vi "Pick&Place_ladder_tang.vi"() -> ()   [LabVIEW 2016]
uses:
  WTF is this.ctl
  Classes/Controllers/I-O/Copy of NI-DAQ Folder/NI-DAQ.lvclass
  D:/INTT/V1/Classes/Controllers/I-O/Copy of I-O Folder/I-O.lvclass
  Classes/Controllers/Dispenser/Copy of Ultimus V2 Folder/Ultimus V2.lvclass
  <vilib>/Analysis/coordinate.llb/2D Cartesian Coordinate Rotation (Scalar).vi
  <vilib>/Utility/file.llb/Read Delimited Spreadsheet (DBL).vi
  <vilib>/Utility/file.llb/Write Delimited Spreadsheet (DBL).vi
  Classes/Controllers/Motion/Copy of Motion Folder/Motion.lvclass
  Classes/Controllers/Camera/Copy of Controller Folder/Controller.lvclass
  <vilib>/Analysis/NI_AALPro.lvlib
  Classes/Controllers/I-O/Copy of I-O Folder/I-O.lvclass
panel:
  out "HDI center positions":dbl[][](array[numeric])=[[459.92445114002015, 980.2358762511564, 78.77350133595746, 0.0015214873297426886]]
  out "x+y":dbl[](array[numeric])
  in  "pick &place module":i32=1
  in  "txt switch":bool
  in  "offset":dbl[][](array[numeric])=[[0.0, 0.0, 0.0, 0.0], [0.0, 0.0, 0.0, 0.0]]
  out "HPoS_CT":dbl[][](array[numeric]) format="%#_8g"
  out "chip distance by OGP":dbl format="%#_8g"
  out "displacement":dbl[](array[numeric])
  out "gantry position test":dbl[](array[numeric])
  out "stave target position":dbl[](array[numeric])
  out "chip distance by gantry":dbl format="%#_8g"
  out "after SL":dbl[](array[numeric]) format="%#_8g"
  out "after SR":dbl[](array[numeric]) format="%#_8g"
  out "after NL":dbl[](array[numeric]) format="%#_8g"
  out "S chip":dbl[](array[numeric]) format="%#_8g"
  out "N chip":dbl[](array[numeric]) format="%#_8g"
  in  "file path (dialog if empty) 2":path=path "C:/Users/PAGANIS/Desktop/shih cheng wei/OGP/test1-2.txt"
  out "bless from OGP !!! Center of  stave":dbl[](array[numeric])
  out "bless from OGP !! measured stave size":dbl[](array[numeric])
  in  "Bless from OGP":bool
  out "FROM Detail !!! Center of module on stave":dbl[](array[numeric])
  out "FROM Detail !! measured stave size":dbl[](array[numeric])
  in  "Align Stave in detail":bool
  in  "check height?":bool
  in  "Uttimus presssure":i64=10
  out "Status":bool
  out "measured HDI top-left position":dbl[][](array[numeric])
  in  "HDI vacuum channel":i32=18
  in  "vacuum":bool=TRUE
  in  "HDI vacuum":bool
  out "measured stave size":dbl[](array[numeric])
  out "Stave mark":dbl[][](array[numeric])
  out "Center of module on stave":dbl[](array[numeric])
  out "Center of HDI from alignment mark":dbl[](array[numeric])
  out "Measured HDI size":dbl[][](array[numeric])
  out "module positions on stave":T1[][](array[typedef])
  in  "Default Stave dimension":dbl[](array[numeric])=[34.0, 472.0, -0.335295, -0.000320234]
  in  "Default Stave upper left mark":dbl[](array[numeric])=[584.376, 675.576, 70.9882, 0.000840064]
  out "Needle parking position":dbl[](array[numeric])
  in  "Uppler / Lower Stave":bool=TRUE
  out "Gantry current position":dbl[](array[numeric])
  in  "READ Position":bool
  in  "Needle Height Compenstation\n(glue gap)":dbl=0.33
  in  "Needle Alignment":bool
  in  "Parking position":dbl[](array[numeric])=[625.0, 625.0, 0.0, 0.01]
  in  "GOTO":bool
  in  "Default Pickup Tool Position":dbl[][](array[numeric])=[[152.226, 682.729, 36.8129, -0.0151898], [700.0, 800.0, 20.0, 0.01]]
  in  "deposit glue module":i32=1
  in  "Default HDI alignment \nmark position":dbl[](array[numeric])=[448.322, 976.582, 74.9872, 0.000191129]
  in  "Default HDI size":dbl[](array[numeric])=[24.2437, 231.446, -0.099339, 0.000191129]
  out "# of tasks excuted":i32
  out "PickupTool \nCenterPosition":dbl[](array[numeric])
  in  "Inititalize":bool
  in  "Pick and place":bool
  in  "Deposit Glue":bool
  in  "Measure Pickup Tools":bool
  in  "Align Stave":bool
  out "default module position on stave":dbl[][](array[numeric])
  in  "Stop":bool
  in  "Measure HDI":bool
  # "Ladder Assembly"
  # "Lower\nmodule"
  # "Upper\nmodule"
  # "+"
  # "="
  # "Sensor 0.32 -> 200 micron glue thickness\nChips 0.37-> 140 micron glue thickness"
  # "ACTIONS"
  # "Stave infomation"
  # "also to switch Upper/Lower"
  # "theta had *-1"
  # "Module infomation"
  # "Pick and Place"
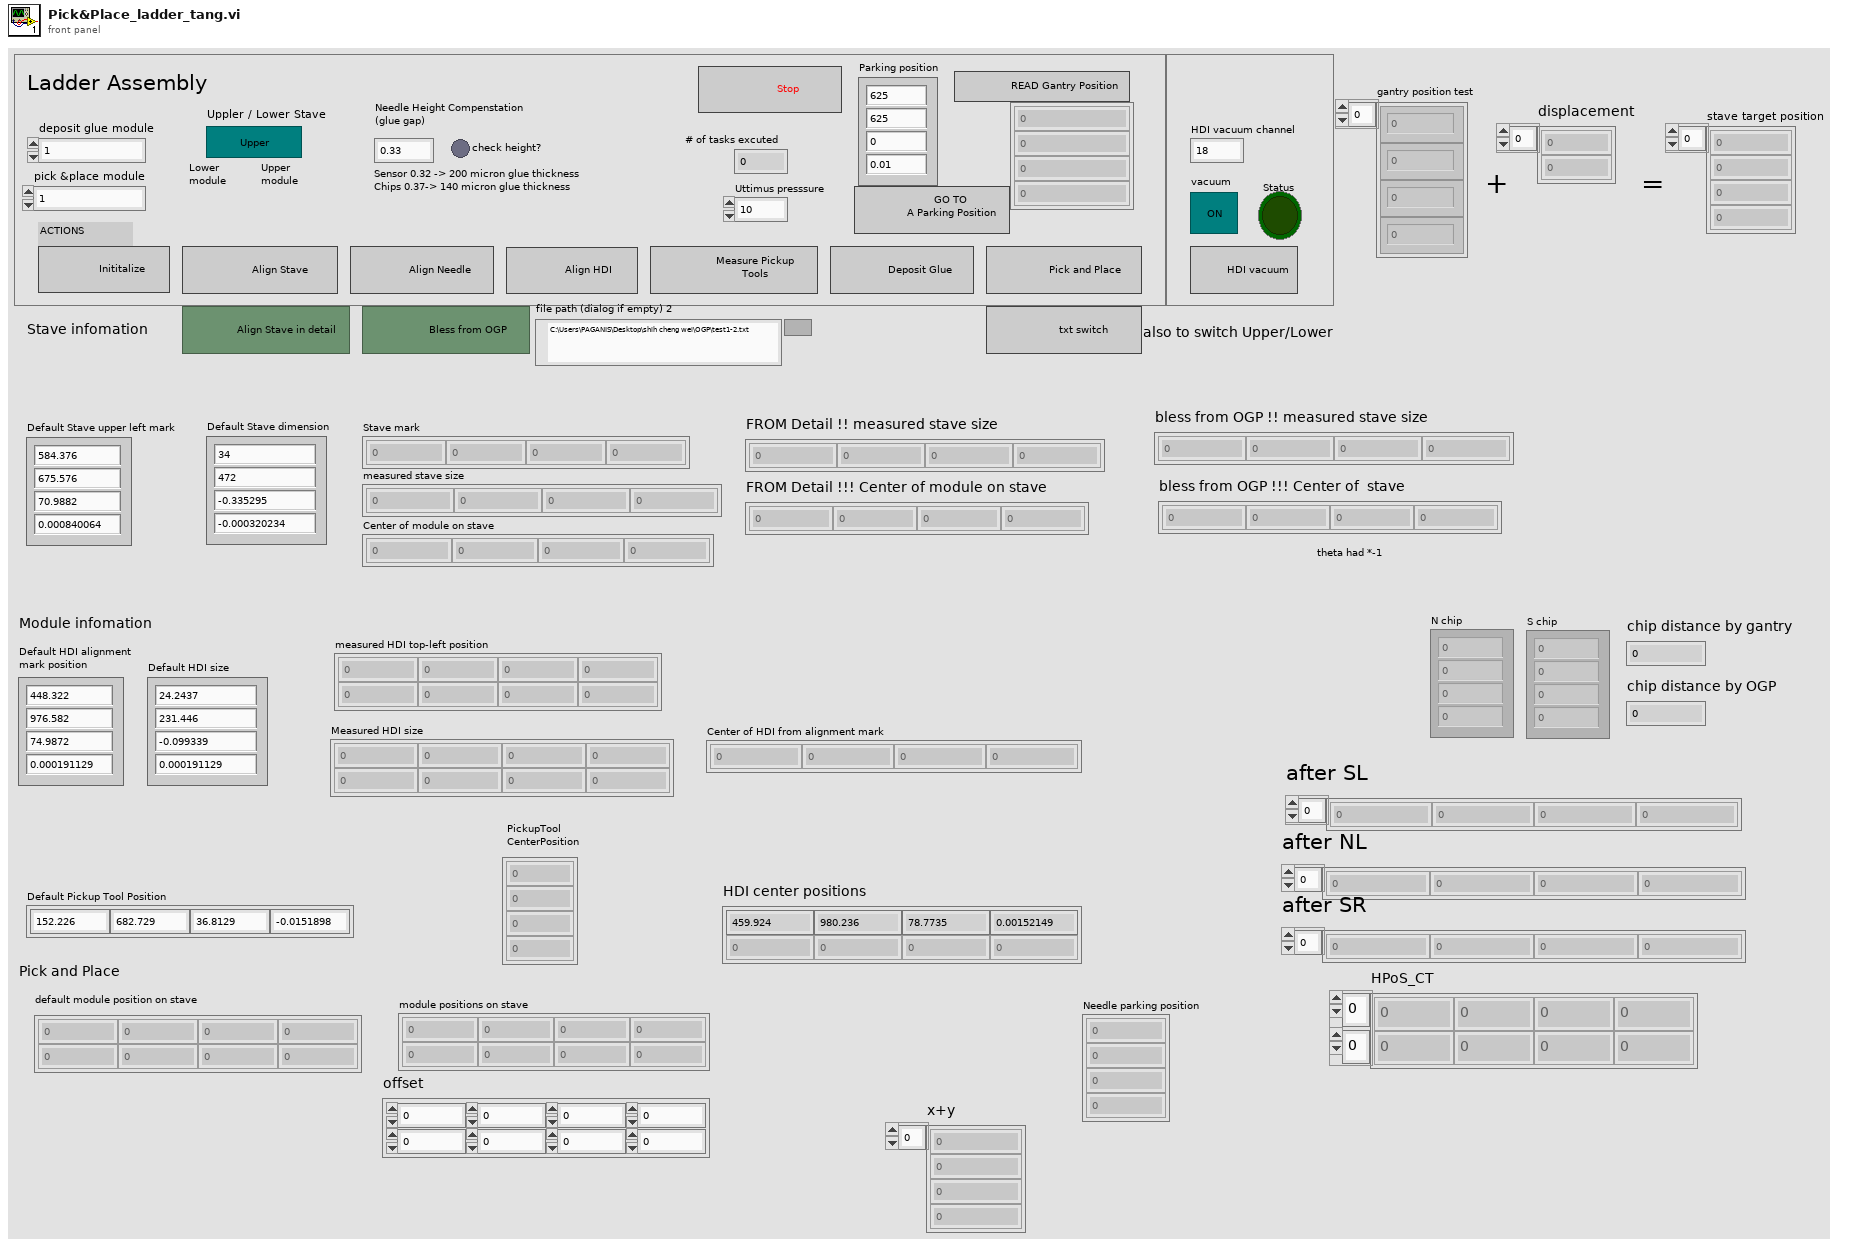
[diagram p1: front panel]
types:
  T1 = typedef "WTF is this.ctl" = dbl
  T2 = typedef "Controller.lvclass/Controllers.ctl" = cluster{"Copy of Motion.lvclass":refnum<class "Motion.lvclass">, "Copy of I-O.lvclass":refnum<class "I-O.lvclass">, "Copy of Dispenser.lvclass":refnum<class "Dispenser.lvclass">}
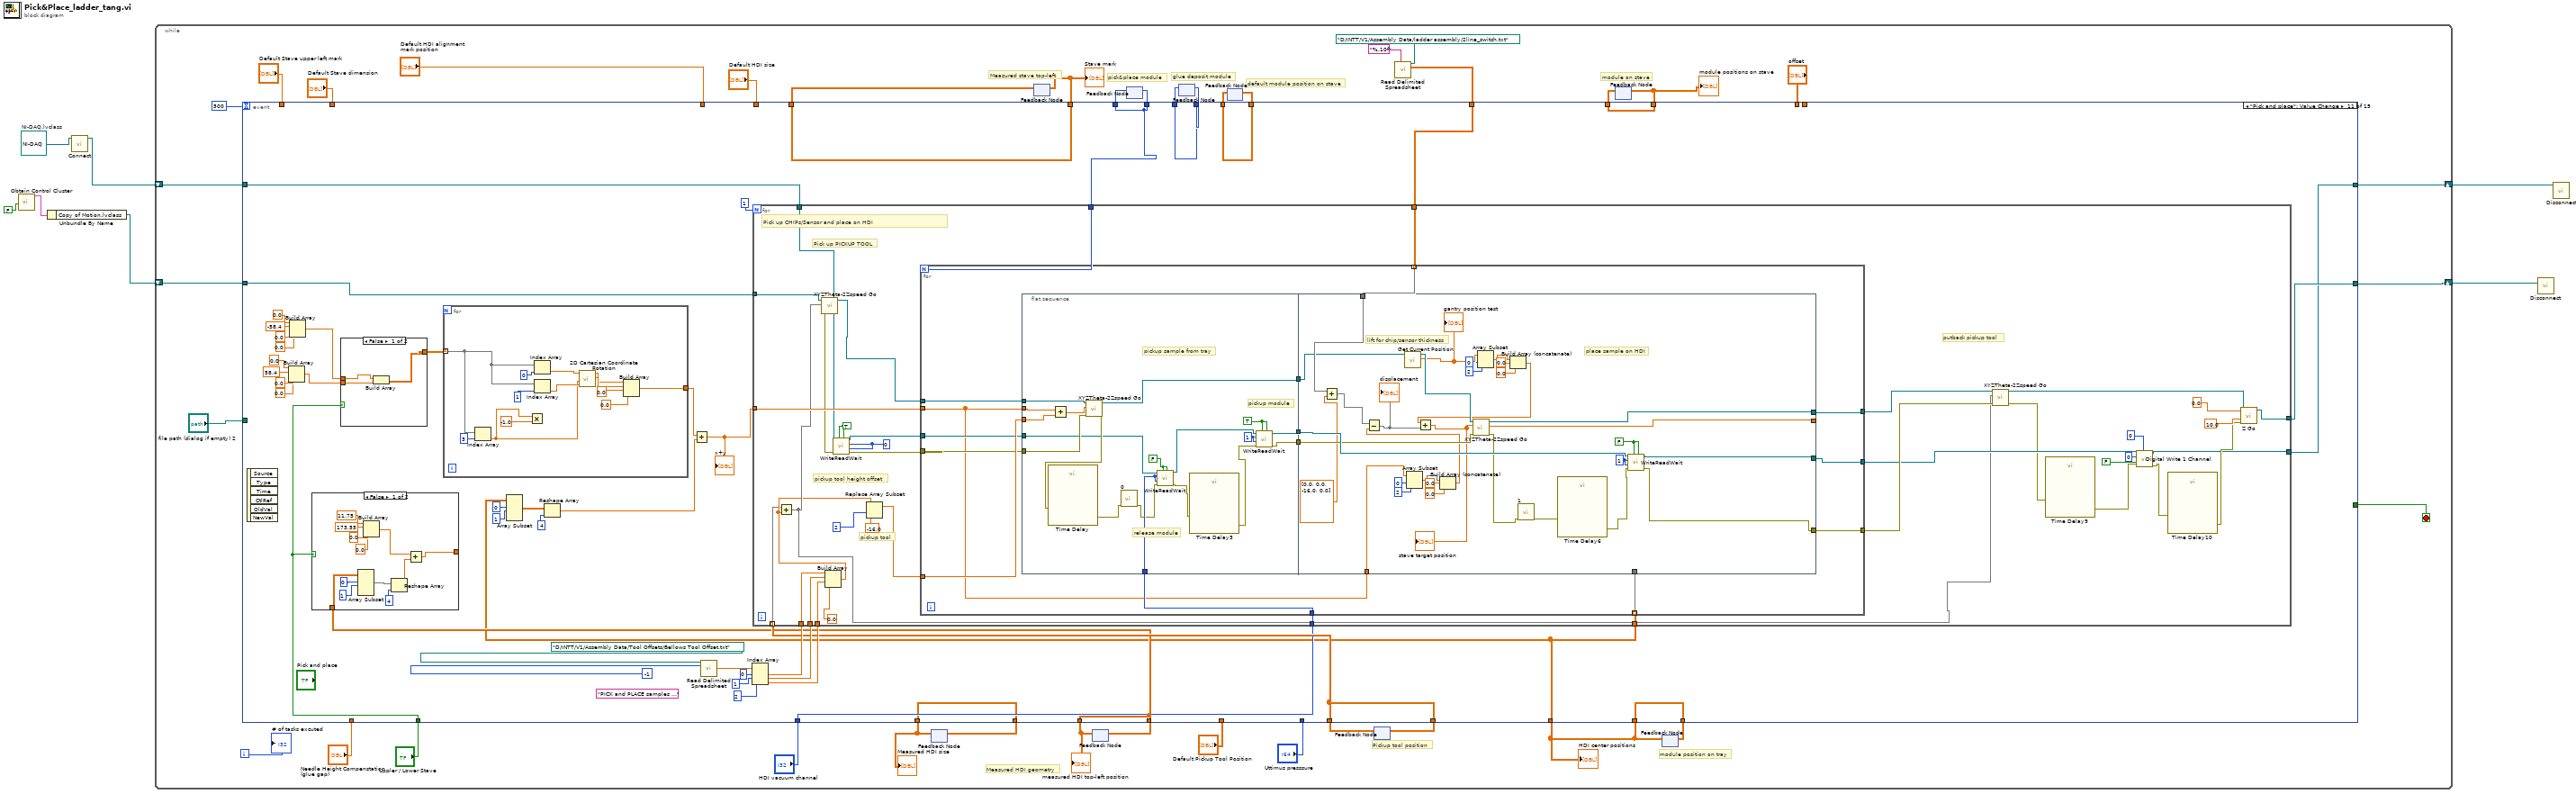
[diagram p0: block diagram]
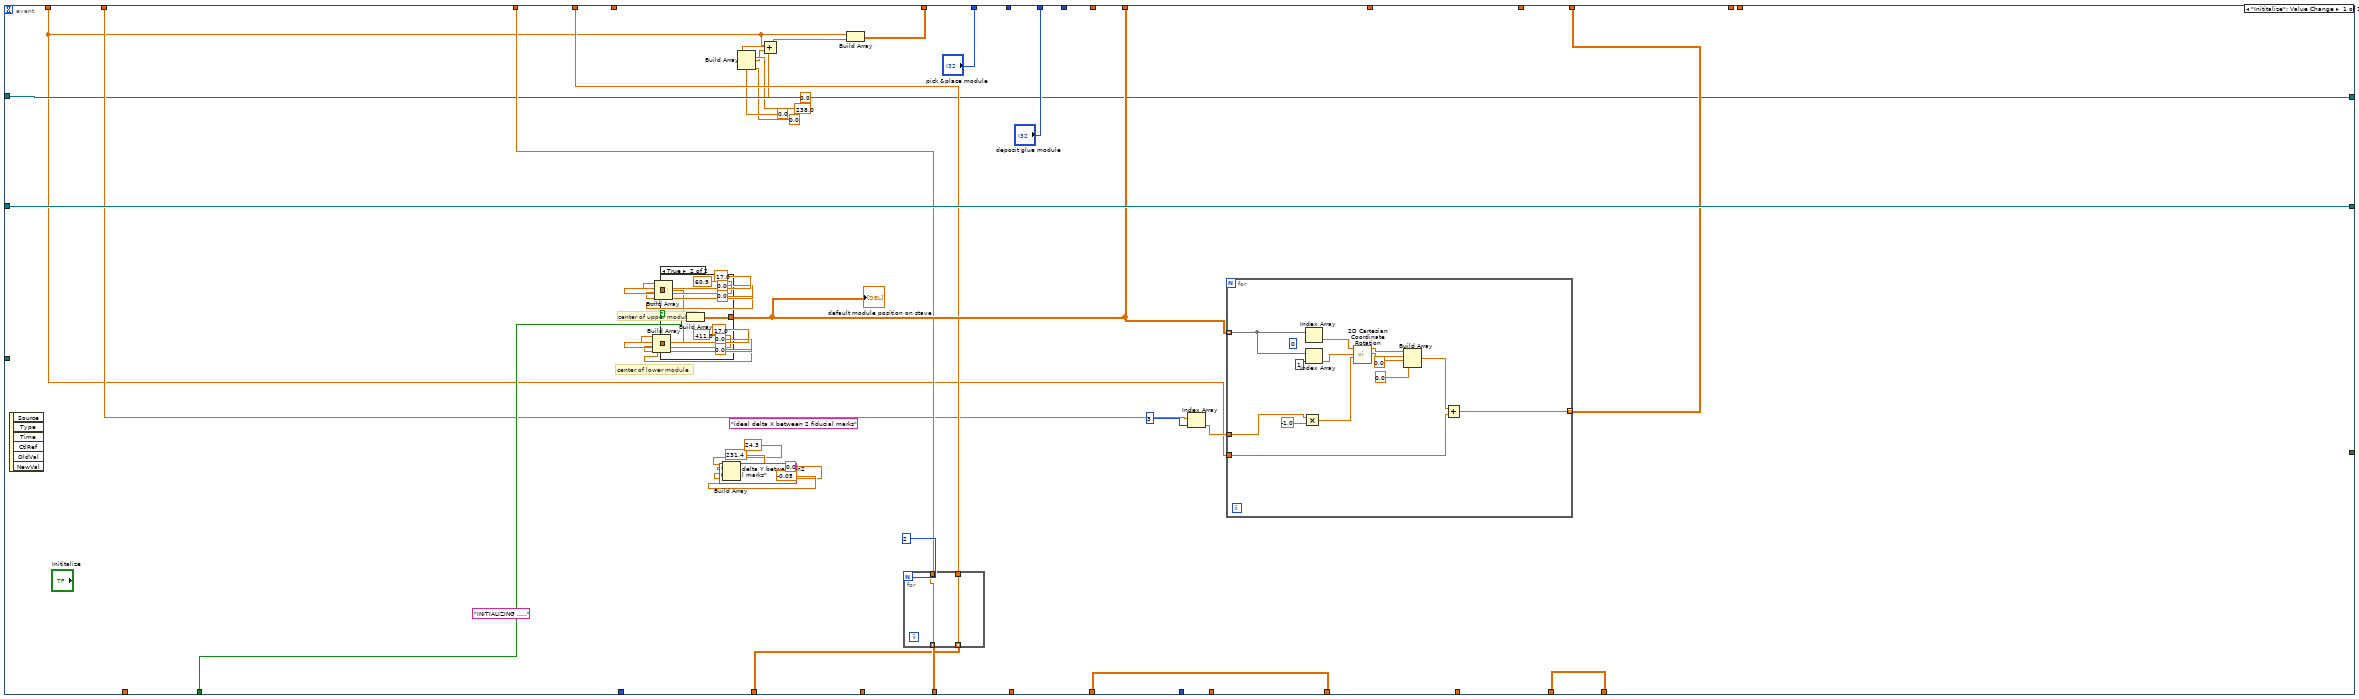
[diagram p2: hidden frame]
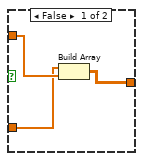
[diagram p3: hidden frame]
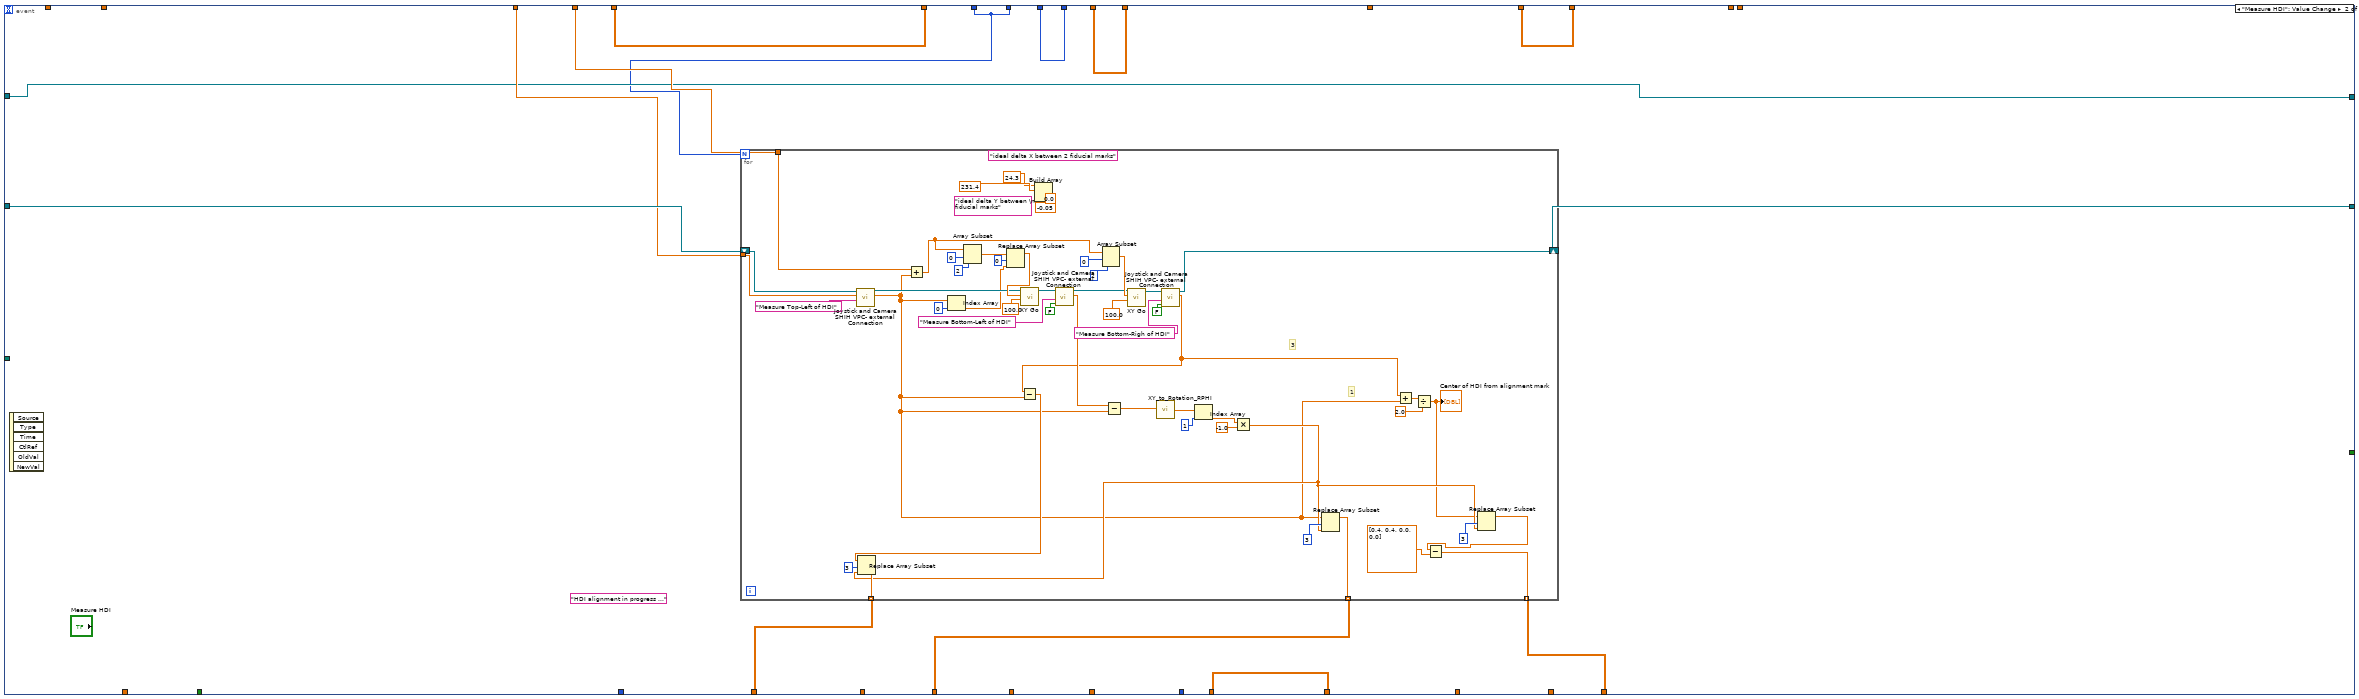
[diagram p4: hidden frame]
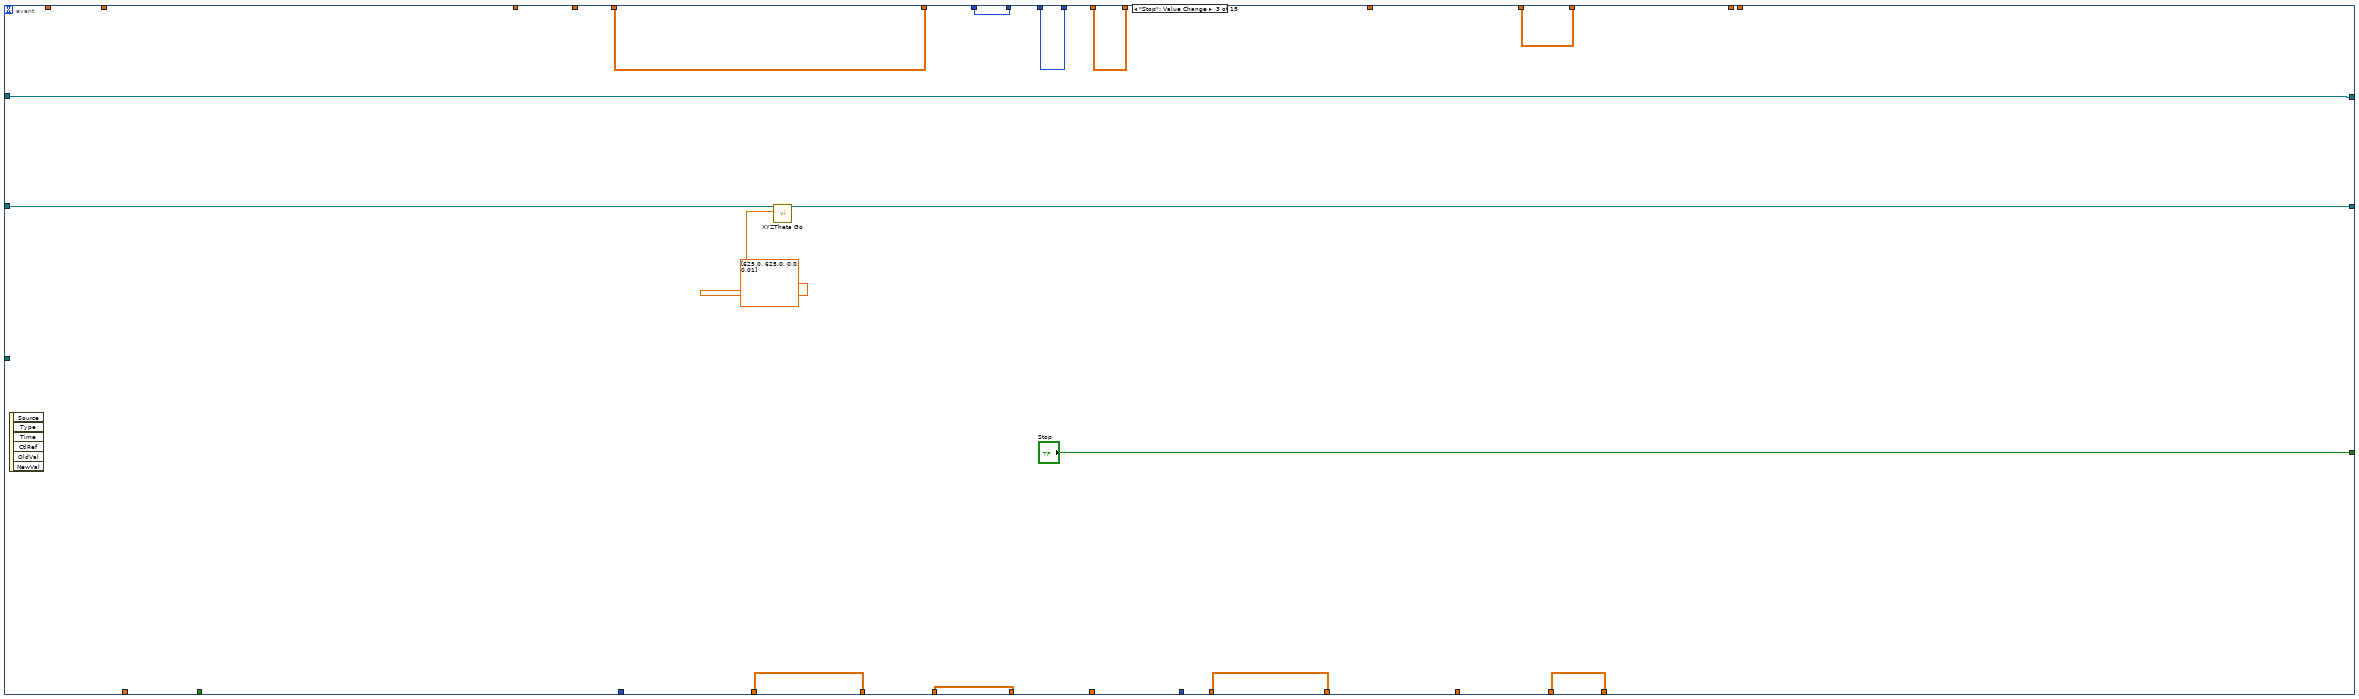
[diagram p5: hidden frame]
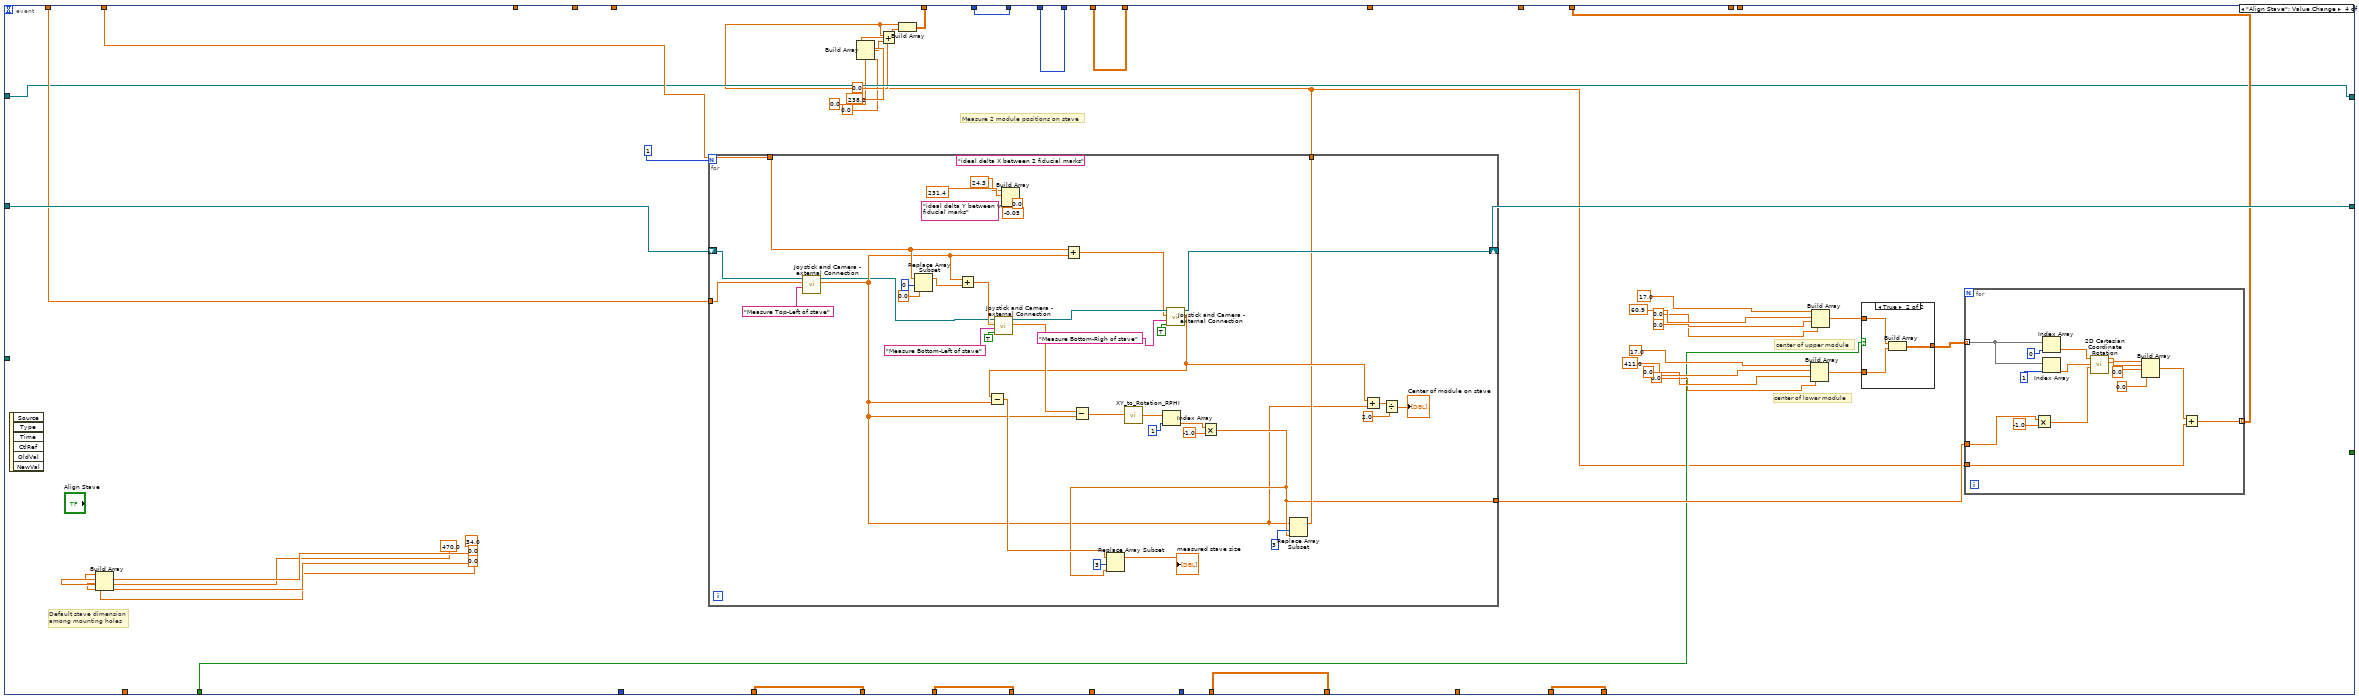
[diagram p6: hidden frame]
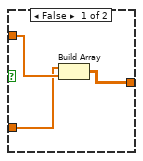
[diagram p7: hidden frame]
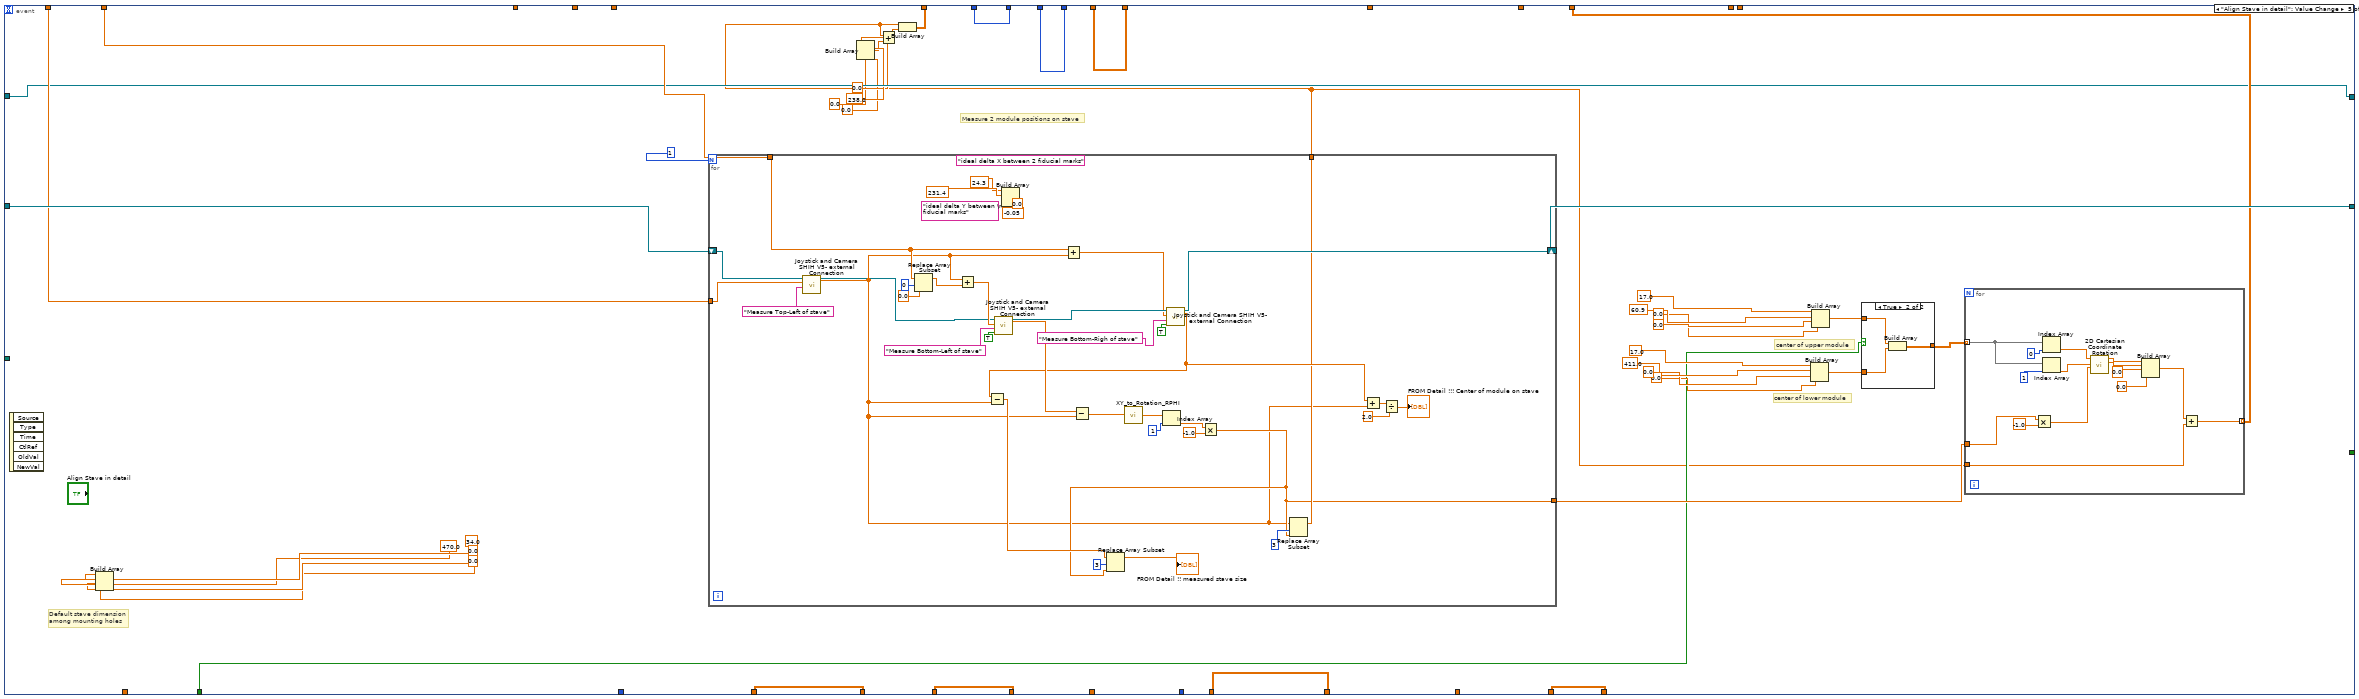
[diagram p8: hidden frame]
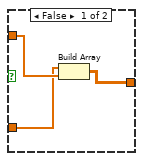
[diagram p9: hidden frame]
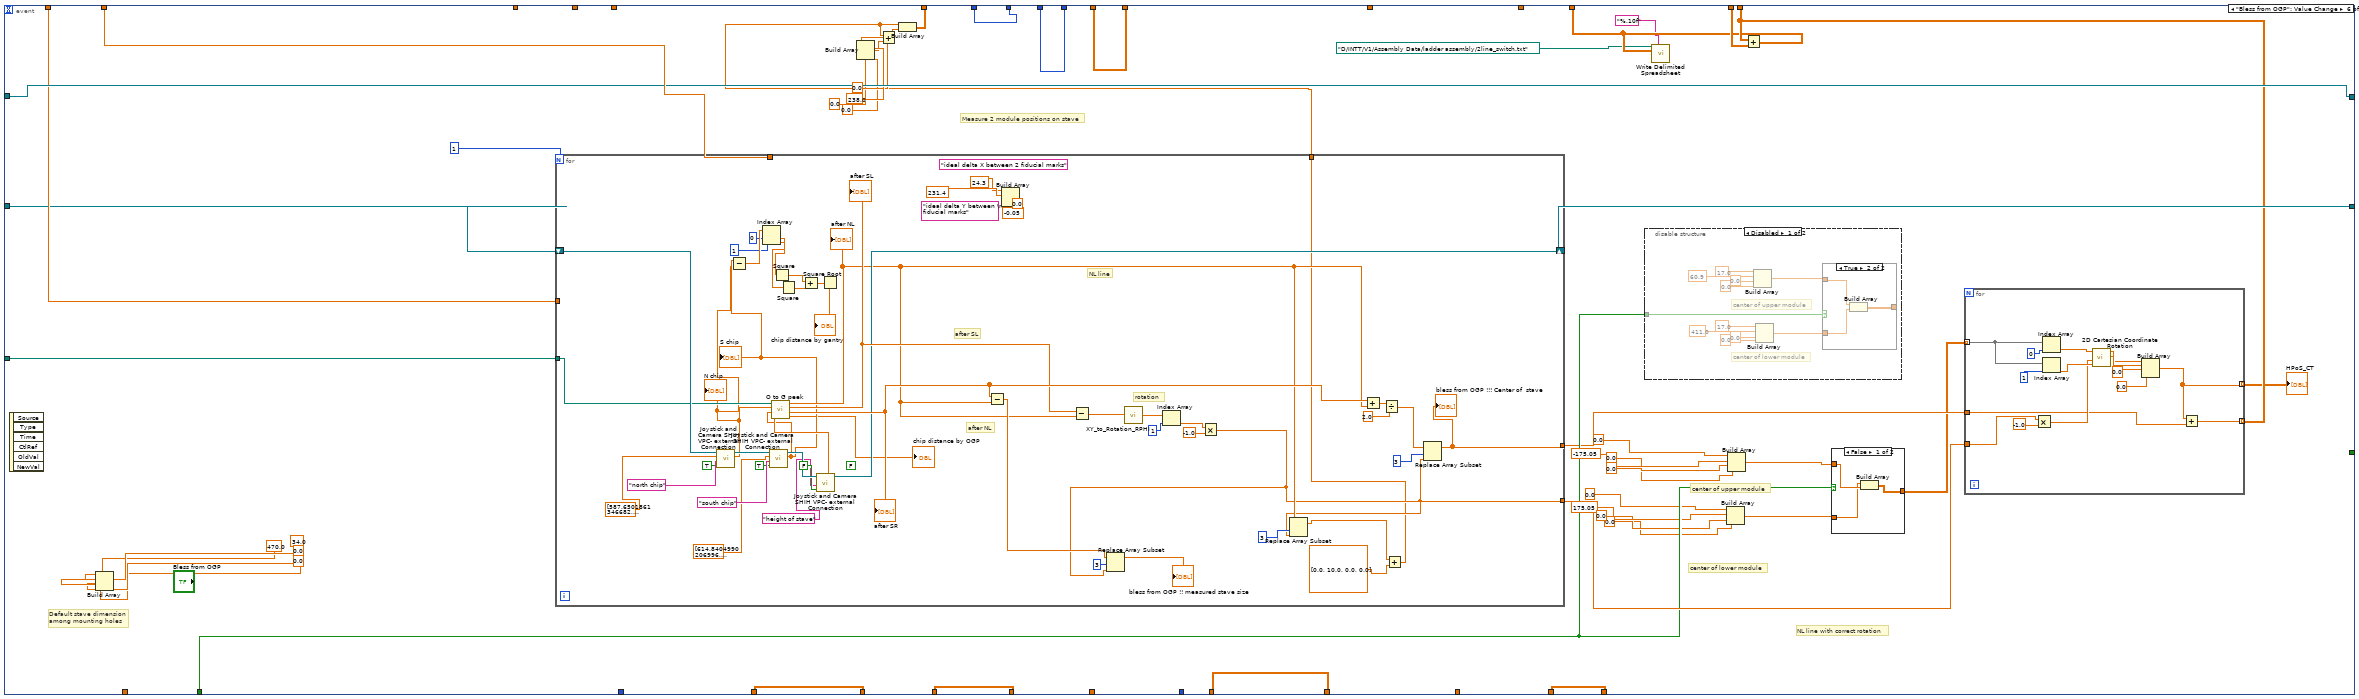
[diagram p10: hidden frame]
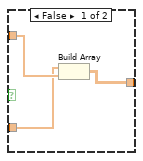
[diagram p11: hidden frame]
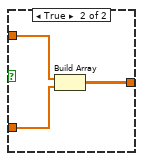
[diagram p13: hidden frame]
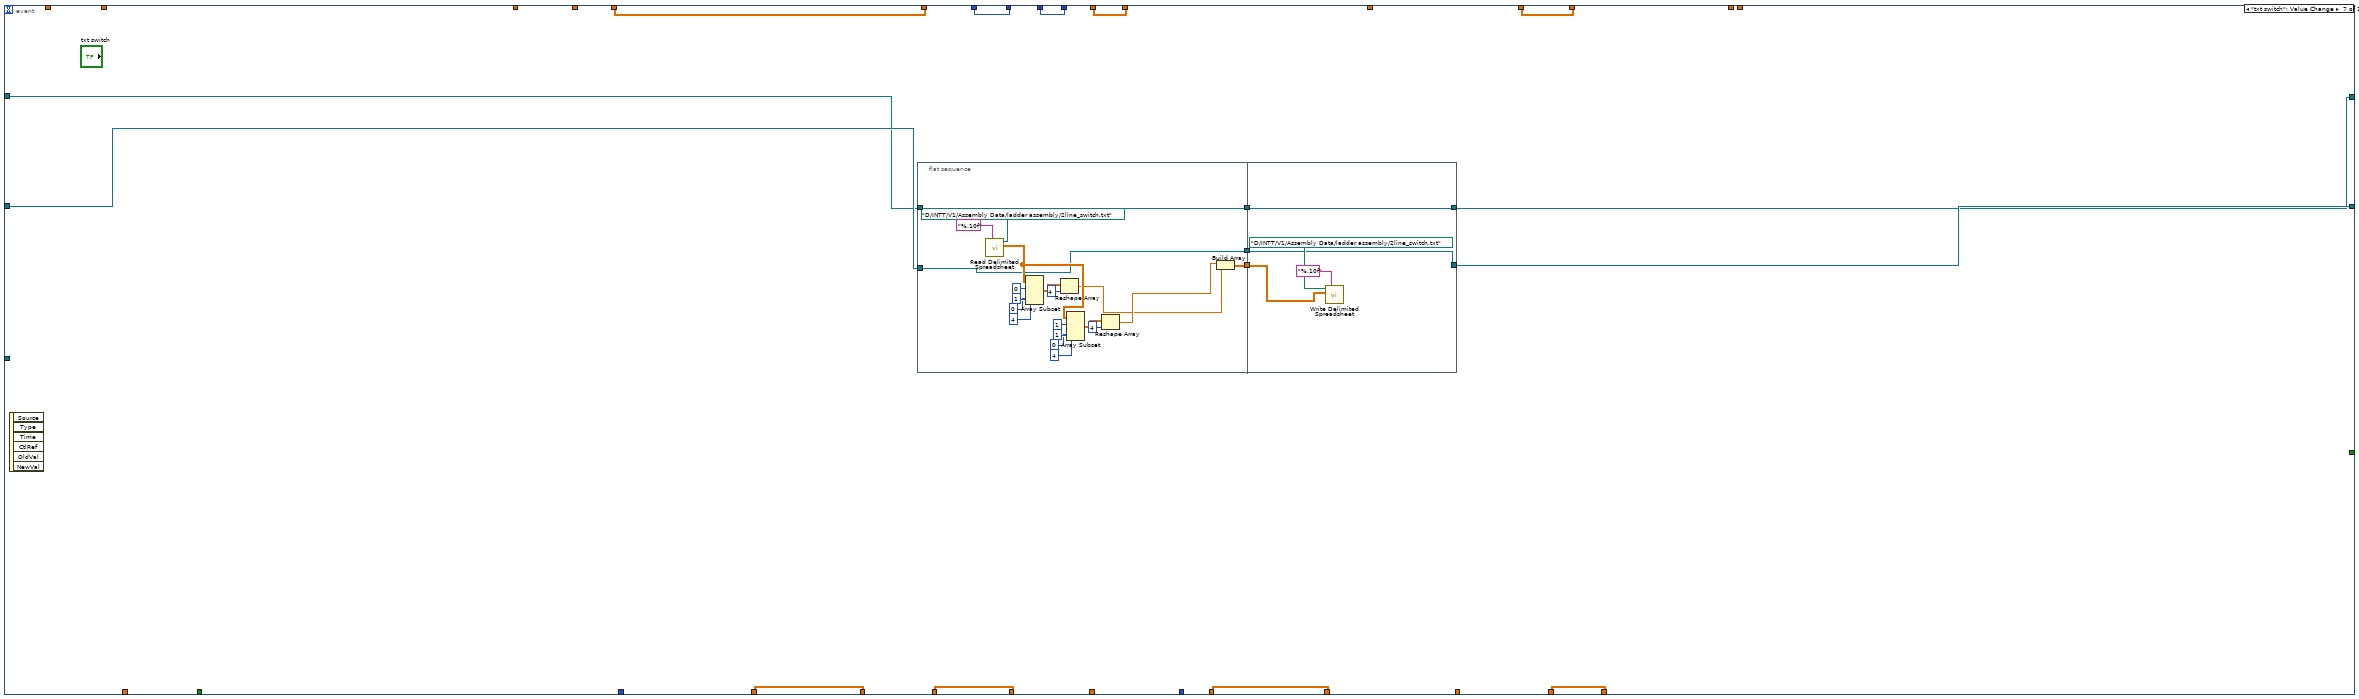
[diagram p14: hidden frame]
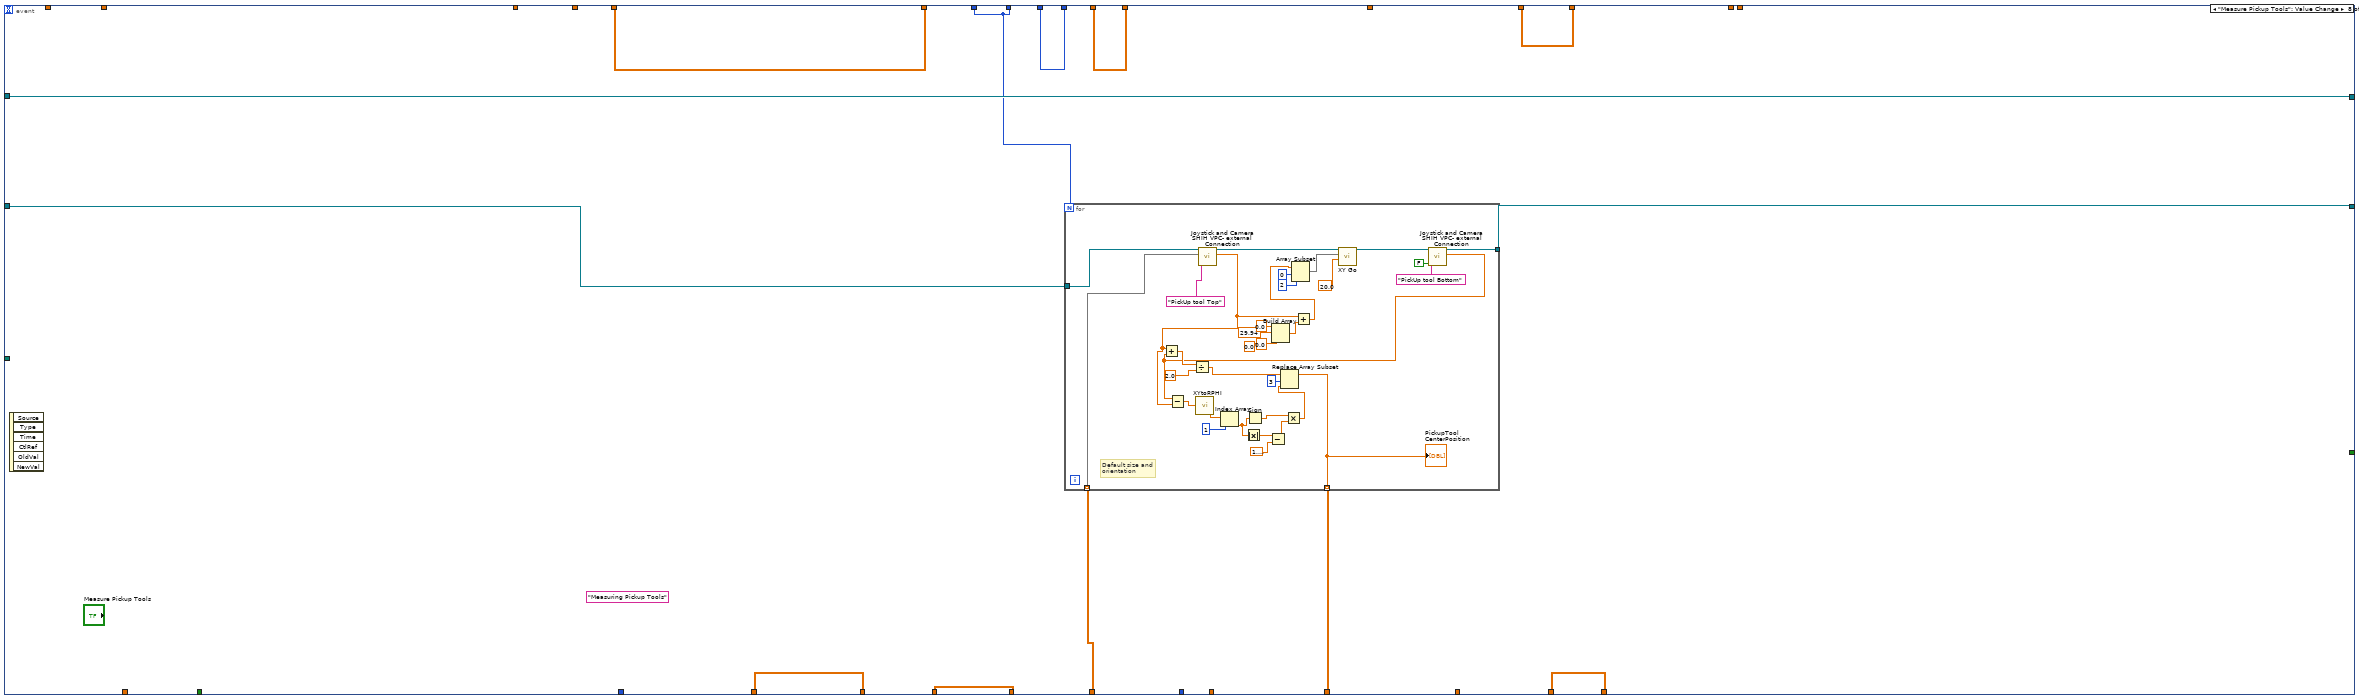
[diagram p15: hidden frame]
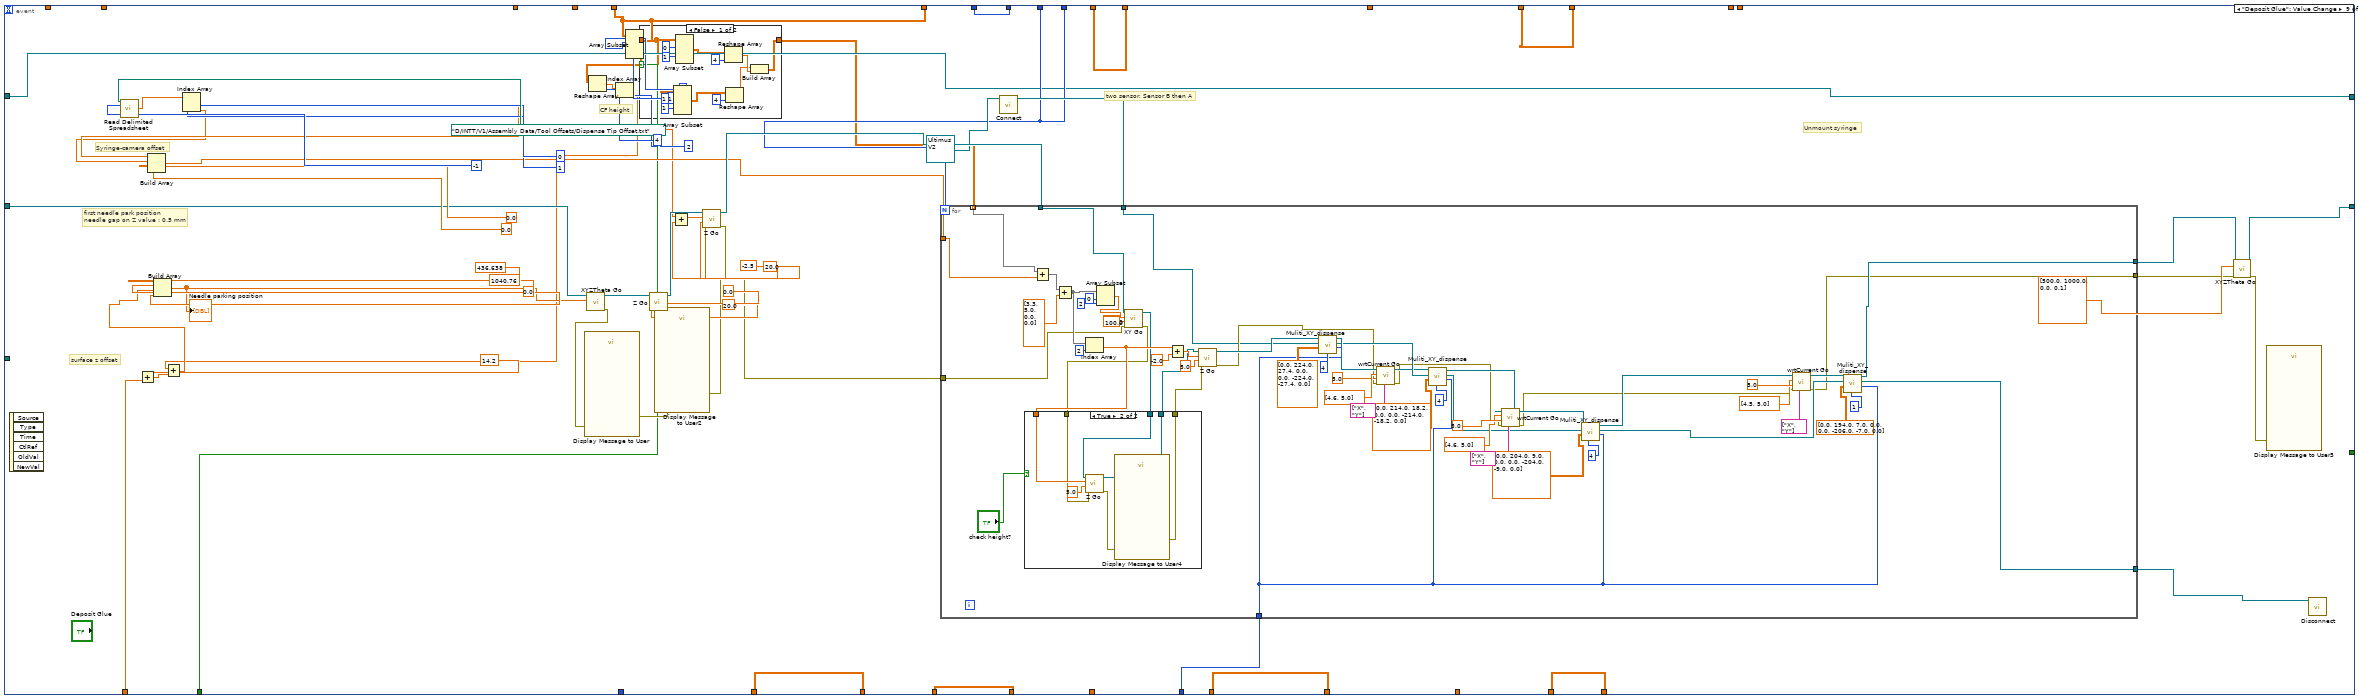
[diagram p16: hidden frame]
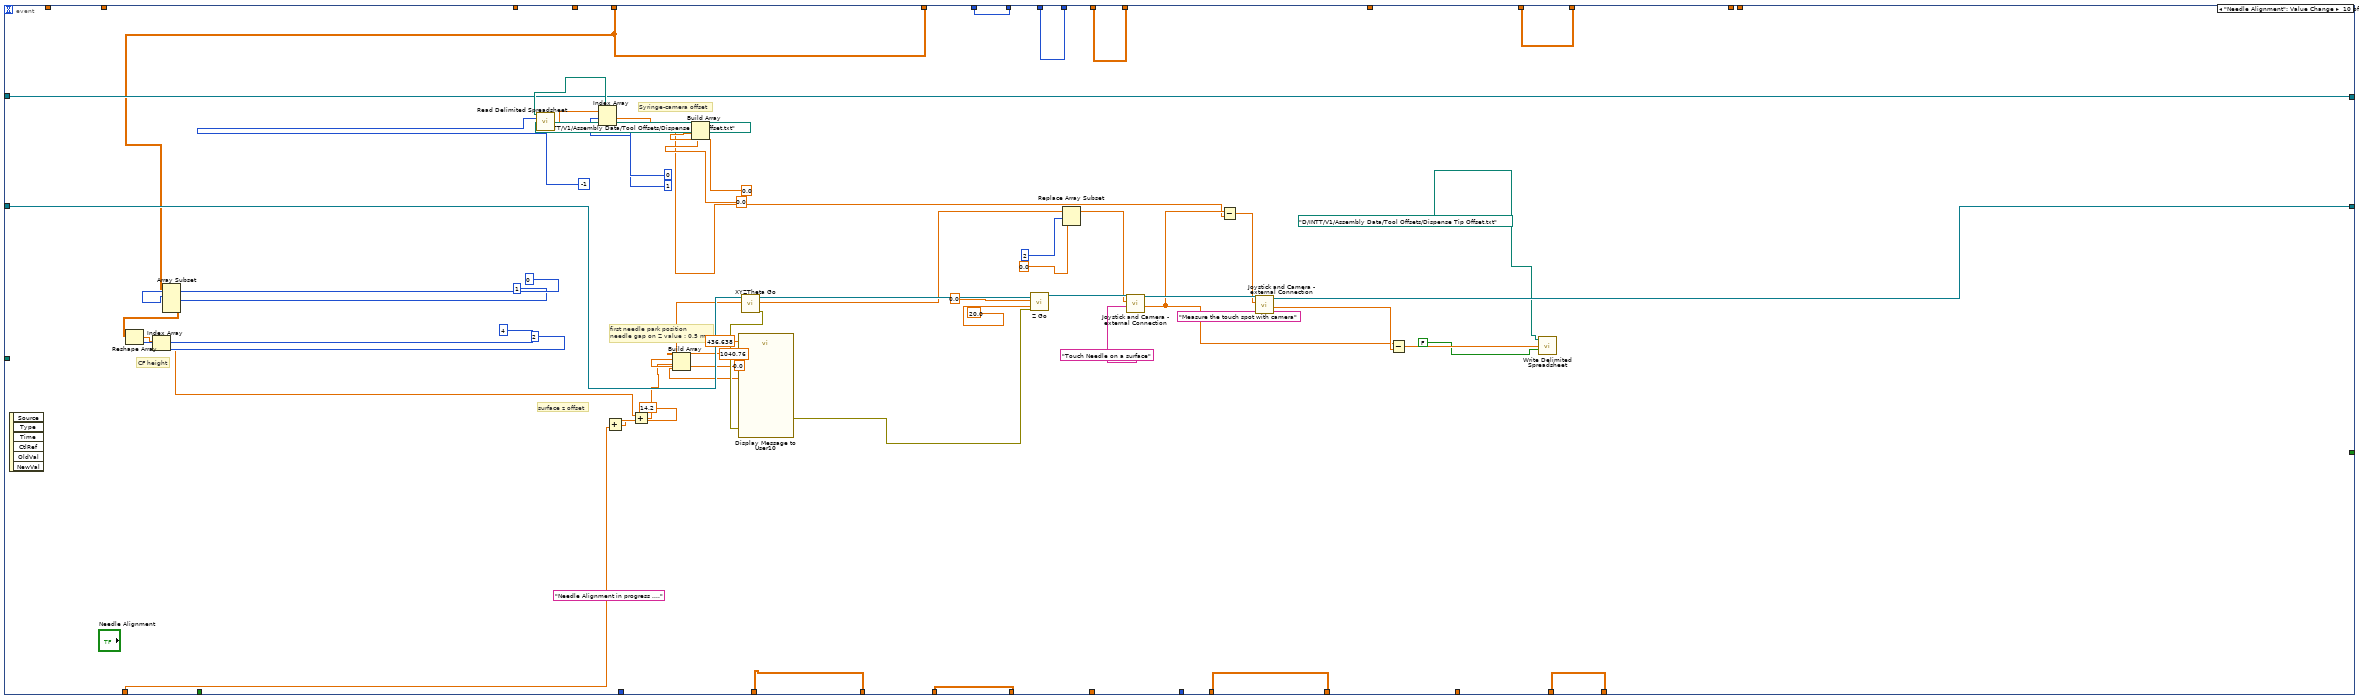
[diagram p19: hidden frame]
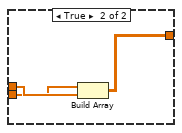
[diagram p20: hidden frame]
diagram:
  w3 = refnum<class "NI-DAQ.lvclass"> refnum  # NI-DAQ.lvclass
  n1 = call "Obtain Control Cluster.vi"("I/O"=FALSE) -> ("Control Out"=w7:T2)  [unwired: 10 in]
  n2 = Unbundle By Name(w7) -> ("Copy of Motion.lvclass"=w5:refnum<class "Motion.lvclass">)
  n3 = call-dynamic "Connect.vi"("NI-DAQ in"=w3) -> ("NI-DAQ out"=w2:refnum<class "NI-DAQ.lvclass">)  [unwired: 9 in, 1 out]
  n4 = while {
    shift-right: [w39] -> w4
    shift-left: w5 -> [w46]
    shift-right: [w19] -> w1
    shift-left: w2 -> [w23]
    i -> [w38]
    stop <- w45 stop-if-true
    # "pick&place module"
    # "default module position on stave"
    # "Pickup tool position"
    # "glue deposit module"
    # "Measured HDI geometry"
    # "module position on tray"
    # "Measured stave top-left"
    # "module on stave"
    n5 = feedback #1() -> (w43:dbl[][])  [unwired: 1 in]
    n6 = feedback #2() -> (w44:dbl[][])  [unwired: 1 in]
    n7 = feedback #3() -> (w20:dbl[][])  [unwired: 1 in]
    n8 = feedback #4() -> (w9:i32)  [unwired: 1 in]
    n9 = feedback #5() -> (w37:i32)  [unwired: 1 in]
    n10 = feedback #6() -> (w32:dbl[][])  [unwired: 1 in]
    n11 = feedback #7() -> (w40:dbl[][])  [unwired: 1 in]
    n12 = call-poly <vilib>:"Read Delimited Spreadsheet.vi"("file path (dialog if empty)"=path "D:/INTT/V1/Assembly Data/ladder assembly/2line_switch.txt" ("file path (dialog if empty) 3"), "format (%.3f)"="%.10f") -> ("all rows"=w11:dbl[][])  [unwired: 8 in, 5 out]
    n13 = feedback #8() -> (w27:dbl[][])  [unwired: 1 in]
    n14 = feedback #9() -> (w8:dbl[][])  [unwired: 1 in]
    "HDI center positions" <- w8
    n15 = event shown="[10] \"Pick and place\": Value Change" {
      selector: _ -> [_ _ _ _ _ _ _ _ _ _ _ _ _ _ _]
      dyn-events: _ -> [_ _ _ _ _ _ _ _ _ _ _ _ _ _ _]
      timeout: 500 -> [_ _ _ _ _ _ _ _ _ _ _ _ _ _ _]
      tunnel: w46 -> [w81 w121 w186 w217 w314 w401 w521 w569 w643 w778 w842 w995 w1014 w1017 w1039]
      tunnel: [_ _ "Stop" _ _ _ _ _ _ _ _ _ _ _ _] -> w45
      tunnel: [w48 w115 w181 w188 w285 w404 w526 w564 w605 w744 w823 w1001 w1010 w1025 w1038] -> w24
      tunnel: w44 -> [_ w115 w181 _ _ _ w526 w564 w605 w744 w823 w1001 w1010 w1025 w1038]
      tunnel: [w58 w113 w180 w213 w310 w416 w530 w563 w629 w781 w825 w998 w1009 w1019 w1036] -> w25
      tunnel: w43 -> [_ _ w180 w213 w310 w416 w530 w563 w629 w781 w825 w998 w1009 w1019 w1036]
      tunnel: w37 -> [_ w108 w183 w218 w315 w419 w525 w560 w632 w783 w819 w1000 w1011 w1023 w1030]
      tunnel: [w63 w112 w178 w220 w317 w421 w527 w562 w631 w779 w808 w996 w1007 w1021 w1033] -> w42
      tunnel: w8 -> [w63 _ w178 w220 w317 w421 w527 w562 w631 w779 w808 w996 w1007 w1021 w1033]
      tunnel: [w79 w116 w179 w225 w322 w426 w528 w568 w630 w780 w831 w997 w1008 w1020 w1034] -> w41
      tunnel: w40 -> [_ w116 w179 w225 w322 w426 w528 _ w630 w780 w831 w997 w1008 w1020 w1034]
      tunnel: [w81 w120 w184 w214 w311 w417 w519 w567 w633 w770 w832 w993 w1013 w1017 w1039] -> w39
      tunnel: ["deposit glue module" w108 w183 w218 w315 w419 w525 w560 w632 w783 w819 w1000 w1011 w1023 w1030] -> w36
      tunnel: "Default HDI alignment \nmark position" -> [w61 w119 _ _ _ _ _ _ _ _ _ _ _ _ _]
      tunnel: "Default HDI size" -> [w60 w118 _ _ _ _ _ _ _ _ _ _ _ _ _]
      tunnel: [w68 w117 w182 w219 w316 w420 w524 w565 w628 w782 w830 w999 w1012 w1024 w1037] -> w33
      tunnel: w32 -> [_ w117 w182 w219 w316 w420 w524 w565 w628 w782 w830 w999 w1012 w1024 w1037]
      tunnel: "Default Pickup Tool Position" -> [w79 _ _ _ _ _ _ w566 _ _ _ _ _ _ _]
      tunnel: "Uppler / Lower Stave" -> [w64 _ _ w198 w295 w399 _ _ w613 _ w818 _ _ _ _]
      tunnel: "Default Stave upper left mark" -> [w49 _ _ w216 w313 w403 _ _ _ _ _ _ _ _ _]
      tunnel: "Default Stave dimension" -> [w57 _ _ w215 w312 w418 _ _ _ _ _ _ _ _ _]
      tunnel: [w65 w114 w176 w197 w294 w384 w523 w561 w627 w761 w821 w991 w1004 w1022 w1032] -> w26
      tunnel: w27 -> [_ w114 w176 _ _ _ w523 w561 w627 w761 w821 w991 w1004 w1022 w1032]
      tunnel: w23 -> [w56 w110 w174 w196 w293 w412 w518 w558 w622 w759 w828 w990 w1003 w1029 w1042]
      tunnel: [w56 w110 w174 w196 w293 w412 w516 w558 w622 w759 w827 w990 w1003 w1016 w1040] -> w19
      tunnel: "HDI vacuum channel" -> [_ _ _ _ _ _ _ _ _ _ w826 _ _ w1026 w1041]
      tunnel: [w59 w111 w175 w212 w309 w415 w529 w559 w623 w760 w824 w992 w1005 w1018 w1035] -> w21
      tunnel: w20 -> [_ _ w175 w212 w309 w415 w529 w559 w623 w760 w824 w992 w1005 w1018 w1035]
      tunnel: "Needle Height Compenstation\n(glue gap)" -> [_ _ _ _ _ _ _ _ w615 w752 _ _ _ _ _]
      tunnel: "Uttimus presssure" -> [_ _ _ _ _ _ _ _ w614 _ _ _ _ _ _]
      tunnel: "file path (dialog if empty) 2" -> [_ _ _ _ _ w402 _ _ _ _ _ _ _ _ _]
      tunnel: [_ _ _ _ _ w400 _ _ _ _ _ _ _ _ _] -> _
      tunnel: "offset" -> [_ _ _ _ _ w385 _ _ _ _ _ _ _ _ _]
      tunnel: w11 -> [_ _ _ _ _ _ _ _ _ _ w822 _ _ _ _]
      tunnel: ["pick &place module" w109 w173 w187 w284 w381 w522 w557 w604 w742 w820 w989 w1002 w1015 w1031] -> w10
      tunnel: w9 -> [_ w109 w173 w187 w284 w381 w522 w557 w604 w742 w820 w989 w1002 w1015 w1031]
      tunnel: w8 -> [_ _ _ _ _ _ _ _ _ _ w799 _ _ _ _]
      event "Inititalize": Value Change {
        (unwired) "INITIALIZING ....." ("String")
        (unwired) "ideal delta Y between \n2 fiducial marks"
        (unwired) "ideal delta X between 2 fiducial marks"
        # "center of lower module"
        # "center of upper module"
        n16 = event-data() -> ()  [unwired: 1 in, 6 out]
        n17 = Build Array(17.0 ("element"), 411.0 ("element"), 0.0 ("element"), 0.0 ("element")) -> (w69:dbl[])
        n18 = Build Array(17.0 ("element"), 60.9 ("element"), 0.0 ("element"), 0.0 ("element")) -> (w70:dbl[])
        n19 = case shown="True" w64 {
          tunnel: w70 -> [w90 w93]
          tunnel: w69 -> [w89 w92]
          tunnel: [w88 w91] -> w68
          frame False {
            n20 = Build Array(w89, w90) -> (w88:dbl[][])
          }
          frame True {
            n21 = Build Array(w93, w92) -> (w91:dbl[][])
          }
        }
        "default module position on stave" <- w68
        n22 = Build Array(24.3 ("y"), 231.4 ("y"), 0.0 ("element"), -0.05 ("element")) -> ()  [unwired: 1 out]
        n23 = Build Array(0.0 ("element"), 238.0 ("element"), 0.0 ("element"), 0.0 ("element")) -> (w51:dbl[])
        n24 = Add(x=w49, y=w51) -> (x+y=w50:dbl[])
        n25 = Build Array(w49, w50) -> (w48:dbl[][])
        n26 = for {
          N: 2 -> [_]
          tunnel: w61 -> [w87]
          tunnel: [w87] -> w59 mode=indexing
          tunnel: w60 -> [w86]
          tunnel: [w86] -> w58 mode=indexing
        }
        n27 = Index Array(array=w57, index=3) -> (element=w66:dbl)
        n28 = for {
          tunnel: w68 -> [w101] mode=indexing
          tunnel: w66 -> [w95]
          tunnel: w49 -> [w100]
          tunnel: [w98] -> w65 mode=indexing
          (unwired) 0 ("index")
          n29 = Multiply(x=w95, y=-1.0) -> (x*y=w96:dbl)
          n30 = Index Array(array=w101) -> (element=w104:dbl)  [unwired: 1 in]
          n31 = Index Array(array=w101, index=1) -> (element=w103:dbl)
          n32 = call-poly <vilib>:"2D Cartesian Coordinate Rotation.vi"("theta"=w96, "y"=w103, "x"=w104) -> ("y out"=w106:dbl, "x out"=w105:dbl)  [unwired: 6 in, 1 out]
          n33 = Build Array(w105, w106, 0.0 ("element"), 0.0 ("element")) -> (w99:dbl[])
          n34 = Add(x=w99, y=w100) -> (x+y=w98:dbl[])
        }
      }
      event "Measure HDI": Value Change {
        (unwired) "HDI alignment in progress ..." ("String")
        n35 = event-data() -> ()  [unwired: 1 in, 6 out]
        n36 = for {
          N: w109 -> [_]
          tunnel: w118 -> [w135]
          shift-right: [w132] -> w120
          shift-left: w121 -> [w133]
          tunnel: w119 -> [w134]
          tunnel: [w169] -> w111 mode=indexing
          tunnel: [w168] -> w113 mode=indexing
          tunnel: [w122] -> w112 mode=indexing
          (unwired) "ideal delta Y between \n2 fiducial marks"
          (unwired) "ideal delta X between 2 fiducial marks"
          # "1"
          # "3"
          n37 = call "Joystick and Camera SHIH VPC- external Connection.vi"("Motion in"=w133, "XYZTheta"=w134, "Measurement Point"="Measure Top-Left of HDI") -> ("Motion out"=w148:refnum<class "Motion.lvclass">, "Sum"=w125:dbl[])  [unwired: 4 in, 2 out]
          n38 = Add(x=w135, y=w125) -> (x+y=w152:dbl[])
          n39 = Index Array(array=w125, index=0) -> (element=w139:dbl)
          n40 = Array Subset(array=w152, index=0, length=2) -> (w151:dbl[])
          n41 = Replace Array Subset(array=w151, new element=w139, index=0) -> (w149:dbl[])
          n42 = call-dynamic "XY Go.vi"("Speed"=100.0, "XY"=w149, "Motion in"=w148) -> ("Motion out"=w156:refnum<class "Motion.lvclass">)  [unwired: 7 in, 1 out]
          n43 = Build Array(24.3 ("y"), 231.4 ("y"), 0.0 ("element"), -0.05 ("element")) -> ()  [unwired: 1 out]
          n44 = call "Joystick and Camera SHIH VPC- external Connection.vi"("Motion in"=w156, "Measurement Point"="Measure Bottom-Left of HDI", "Inital GO"=FALSE) -> ("Motion out"=w147:refnum<class "Motion.lvclass">, "Sum"=w138:dbl[])  [unwired: 4 in, 2 out]
          n45 = Array Subset(array=w152, index=0, length=2) -> (w162:dbl[])
          n46 = Subtract(x=w138, y=w125) -> (x-y=w146:dbl[])
          n47 = call-dynamic "XY Go.vi"("Speed"=100.0, "XY"=w162, "Motion in"=w147) -> ("Motion out"=w166:refnum<class "Motion.lvclass">)  [unwired: 7 in, 1 out]
          n48 = call "XY_to_Rotation_RPHI.vi"("X-Y"=w146) -> ("r-phi"=w142:dbl[])
          n49 = call "Joystick and Camera SHIH VPC- external Connection.vi"("Motion in"=w166, "Measurement Point"="Measure Bottom-Righ of HDI", "Inital GO"=FALSE) -> ("Motion out"=w132:refnum<class "Motion.lvclass">, "Sum"=w129:dbl[])  [unwired: 4 in, 2 out]
          n50 = Subtract(x=w129, y=w125) -> (x-y=w130:dbl[])
          n51 = Index Array(array=w142, index=1) -> (element=w136:dbl)
          n52 = Multiply(x=w136, y=-1.0) -> (x*y=w127:dbl)
          n53 = Replace Array Subset(array=w130, new element=w127, index=3) -> (w168:dbl[])
          n54 = Replace Array Subset(array=w125, new element=w127, index=3) -> (w169:dbl[])
          n55 = Add(x=w129, y=w125) -> (x+y=w171:dbl[])
          n56 = Divide(x=w171, y=2.0) -> (x/y=w126:dbl[])
          "Center of HDI from alignment mark" <- w126
          n57 = Replace Array Subset(array=w126, new element=w127, index=3) -> (w123:dbl[])
          n58 = Subtract(x=w123, y=dbl[] [0.4, 0.4, 0.0, 0.0]) -> (x-y=w122:dbl[])
        }
      }
      event "Stop": Value Change {
        n59 = event-data() -> ()  [unwired: 1 in, 6 out]
        n60 = call "XYZTheta Go.vi"("XYZTheta In"=dbl[] [625.0, 625.0, 0.0, 0.01], "Motion in"=w186) -> ("Motion out"=w184:refnum<class "Motion.lvclass">)  [unwired: 7 in, 2 out]
      }
      event "Align Stave": Value Change {
        # "center of lower module"
        # "center of upper module"
        # "Default stave dimension\namong mounting holes"
        # "Measure 2 module positions on stave"
        n61 = event-data() -> ()  [unwired: 1 in, 6 out]
        n62 = Build Array(34.0 ("element"), 470.0 ("element"), 0.0 ("element"), 0.0 ("element")) -> ()  [unwired: 1 out]
        n63 = for {
          N: 1 -> [_]
          tunnel: w215 -> [w232]
          shift-right: [w242] -> w214
          shift-left: w217 -> [w243]
          tunnel: w216 -> [w244]
          tunnel: [w237] -> w190
          tunnel: [w235] -> w200
          (unwired) "ideal delta Y between \n2 fiducial marks"
          (unwired) "ideal delta X between 2 fiducial marks"
          n64 = call "Joystick and Camera - external Connection.vi"("Motion in"=w243, "XYZTheta"=w244, "Measurement Point"="Measure Top-Left of stave") -> ("Motion out"=w226:refnum<class "Motion.lvclass">, "Sum"=w228:dbl[])  [unwired: 4 in, 2 out]
          n65 = Replace Array Subset(array=w232, new element=0.0 ("new element/subarray"), index=0) -> (w229:dbl[])
          n66 = Add(x=w228, y=w229) -> (x+y=w227:dbl[])
          n67 = call "Joystick and Camera - external Connection.vi"("Motion in"=w226, "XYZTheta"=w227, "Measurement Point"="Measure Bottom-Left of stave", "Inital GO"=TRUE) -> ("Motion out"=w234:refnum<class "Motion.lvclass">, "Sum"=w247:dbl[])  [unwired: 3 in, 2 out]
          n68 = Build Array(24.3 ("y"), 231.4 ("y"), 0.0 ("element"), -0.05 ("element")) -> ()  [unwired: 1 out]
          n69 = Add(x=w232, y=w228) -> (x+y=w233:dbl[])
          n70 = Subtract(x=w247, y=w228) -> (x-y=w253:dbl[])
          n71 = call "XY_to_Rotation_RPHI.vi"("X-Y"=w253) -> ("r-phi"=w249:dbl[])
          n72 = Index Array(array=w249, index=1) -> (element=w245:dbl)
          n73 = call "Joystick and Camera - external Connection.vi"("Motion in"=w234, "XYZTheta"=w233, "Measurement Point"="Measure Bottom-Righ of stave", "Inital GO"=TRUE) -> ("Motion out"=w242:refnum<class "Motion.lvclass">, "Sum"=w239:dbl[])  [unwired: 3 in, 2 out]
          n74 = Subtract(x=w239, y=w228) -> (x-y=w240:dbl[])
          n75 = Multiply(x=w245, y=-1.0) -> (x*y=w235:dbl)
          n76 = Replace Array Subset(array=w240, new element=w235, index=3) -> (→"measured stave size":dbl[])
          n77 = Replace Array Subset(array=w228, new element=w235, index=3) -> (w237:dbl[])
          n78 = Add(x=w239, y=w228) -> (x+y=w261:dbl[])
          n79 = Divide(x=w261, y=2.0) -> (x/y=→"Center of module on stave":dbl[])
        }
        n80 = Build Array(0.0 ("element"), 238.0 ("element"), 0.0 ("element"), 0.0 ("element")) -> (w191:dbl[])
        n81 = Add(x=w190, y=w191) -> (x+y=w189:dbl[])
        n82 = Build Array(w190, w189) -> (w188:dbl[][])
        n83 = Build Array(17.0 ("element"), 411.0 ("element"), 0.0 ("element"), 0.0 ("element")) -> (w202:dbl[])
        n84 = Build Array(17.0 ("element"), 60.9 ("element"), 0.0 ("element"), 0.0 ("element")) -> (w203:dbl[])
        n85 = case shown="True" w198 {
          tunnel: w203 -> [w280 w283]
          tunnel: w202 -> [w279 w282]
          tunnel: [w278 w281] -> w201
          frame False {
            n86 = Build Array(w279, w280) -> (w278:dbl[][])
          }
          frame True {
            n87 = Build Array(w283, w282) -> (w281:dbl[][])
          }
        }
        n88 = for {
          tunnel: w201 -> [w271] mode=indexing
          tunnel: w200 -> [w266]
          tunnel: w190 -> [w270]
          tunnel: [w268] -> w197 mode=indexing
          n89 = Multiply(x=w266, y=-1.0) -> (x*y=w265:dbl)
          n90 = Index Array(array=w271, index=0) -> (element=w274:dbl)
          n91 = Index Array(array=w271, index=1) -> (element=w273:dbl)
          n92 = call-poly <vilib>:"2D Cartesian Coordinate Rotation.vi"("theta"=w265, "y"=w273, "x"=w274) -> ("y out"=w276:dbl, "x out"=w275:dbl)  [unwired: 6 in, 1 out]
          n93 = Build Array(w275, w276, 0.0 ("element"), 0.0 ("element")) -> (w269:dbl[])
          n94 = Add(x=w269, y=w270) -> (x+y=w268:dbl[])
        }
      }
      event "Align Stave in detail": Value Change {
        # "center of lower module"
        # "center of upper module"
        # "Default stave dimension\namong mounting holes"
        # "Measure 2 module positions on stave"
        n95 = event-data() -> ()  [unwired: 1 in, 6 out]
        n96 = Build Array(34.0 ("element"), 470.0 ("element"), 0.0 ("element"), 0.0 ("element")) -> ()  [unwired: 1 out]
        n97 = for {
          N: 1 -> [_]
          tunnel: w312 -> [w329]
          shift-right: [w339] -> w311
          shift-left: w314 -> [w340]
          tunnel: w313 -> [w341]
          tunnel: [w334] -> w287
          tunnel: [w332] -> w297
          (unwired) "ideal delta Y between \n2 fiducial marks"
          (unwired) "ideal delta X between 2 fiducial marks"
          n98 = call "Joystick and Camera SHIH V5- external Connection.vi"("Motion in"=w340, "XYZTheta"=w341, "Measurement Point"="Measure Top-Left of stave") -> ("final out"=w325:dbl[], "Motion out"=w323:refnum<class "Motion.lvclass">)  [unwired: 5 in, 1 out]
          n99 = Replace Array Subset(array=w329, new element=0.0 ("new element/subarray"), index=0) -> (w326:dbl[])
          n100 = Add(x=w325, y=w326) -> (x+y=w324:dbl[])
          n101 = call "Joystick and Camera SHIH V5- external Connection.vi"("Motion in"=w323, "XYZTheta"=w324, "Measurement Point"="Measure Bottom-Left of stave", "Inital GO"=TRUE) -> ("final out"=w344:dbl[], "Motion out"=w331:refnum<class "Motion.lvclass">)  [unwired: 4 in, 1 out]
          n102 = Build Array(24.3 ("y"), 231.4 ("y"), 0.0 ("element"), -0.05 ("element")) -> ()  [unwired: 1 out]
          n103 = Add(x=w329, y=w325) -> (x+y=w330:dbl[])
          n104 = Subtract(x=w344, y=w325) -> (x-y=w350:dbl[])
          n105 = call "XY_to_Rotation_RPHI.vi"("X-Y"=w350) -> ("r-phi"=w346:dbl[])
          n106 = Index Array(array=w346, index=1) -> (element=w342:dbl)
          n107 = call "Joystick and Camera SHIH V5- external Connection.vi"("Motion in"=w331, "XYZTheta"=w330, "Measurement Point"="Measure Bottom-Righ of stave", "Inital GO"=TRUE) -> ("final out"=w336:dbl[], "Motion out"=w339:refnum<class "Motion.lvclass">)  [unwired: 4 in, 1 out]
          n108 = Subtract(x=w336, y=w325) -> (x-y=w337:dbl[])
          n109 = Multiply(x=w342, y=-1.0) -> (x*y=w332:dbl)
          n110 = Replace Array Subset(array=w337, new element=w332, index=3) -> (→"FROM Detail !! measured stave size":dbl[])
          n111 = Replace Array Subset(array=w325, new element=w332, index=3) -> (w334:dbl[])
          n112 = Add(x=w336, y=w325) -> (x+y=w358:dbl[])
          n113 = Divide(x=w358, y=2.0) -> (x/y=→"FROM Detail !!! Center of module on stave":dbl[])
        }
        n114 = Build Array(0.0 ("element"), 238.0 ("element"), 0.0 ("element"), 0.0 ("element")) -> (w288:dbl[])
        n115 = Add(x=w287, y=w288) -> (x+y=w286:dbl[])
        n116 = Build Array(w287, w286) -> (w285:dbl[][])
        n117 = Build Array(17.0 ("element"), 411.0 ("element"), 0.0 ("element"), 0.0 ("element")) -> (w299:dbl[])
        n118 = Build Array(17.0 ("element"), 60.9 ("element"), 0.0 ("element"), 0.0 ("element")) -> (w300:dbl[])
        n119 = case shown="True" w295 {
          tunnel: w300 -> [w377 w380]
          tunnel: w299 -> [w376 w379]
          tunnel: [w375 w378] -> w298
          frame False {
            n120 = Build Array(w376, w377) -> (w375:dbl[][])
          }
          frame True {
            n121 = Build Array(w380, w379) -> (w378:dbl[][])
          }
        }
        n122 = for {
          tunnel: w298 -> [w368] mode=indexing
          tunnel: w297 -> [w363]
          tunnel: w287 -> [w367]
          tunnel: [w365] -> w294 mode=indexing
          n123 = Multiply(x=w363, y=-1.0) -> (x*y=w362:dbl)
          n124 = Index Array(array=w368, index=0) -> (element=w371:dbl)
          n125 = Index Array(array=w368, index=1) -> (element=w370:dbl)
          n126 = call-poly <vilib>:"2D Cartesian Coordinate Rotation.vi"("theta"=w362, "y"=w370, "x"=w371) -> ("y out"=w373:dbl, "x out"=w372:dbl)  [unwired: 6 in, 1 out]
          n127 = Build Array(w372, w373, 0.0 ("element"), 0.0 ("element")) -> (w366:dbl[])
          n128 = Add(x=w366, y=w367) -> (x+y=w365:dbl[])
        }
      }
      event "Bless from OGP": Value Change {
        # "center of lower module"
        # "center of upper module"
        # "NL line with correct rotation"
        # "Default stave dimension\namong mounting holes"
        # "Measure 2 module positions on stave"
        n129 = event-data() -> ()  [unwired: 1 in, 6 out]
        n130 = Build Array(34.0 ("element"), 470.0 ("element"), 0.0 ("element"), 0.0 ("element")) -> ()  [unwired: 1 out]
        n131 = for {
          N: 1 -> [_]
          tunnel: w418 -> [_]
          shift-right: [w472] -> w417
          shift-left: w401 -> [w485]
          tunnel: w403 -> [_]
          tunnel: [w464] -> w406
          tunnel: [w467] -> w414
          tunnel: w402 -> [w474]
          tunnel: [w450] -> w388
          (unwired) FALSE ("Inital GO")
          (unwired) "ideal delta Y between \n2 fiducial marks"
          (unwired) "ideal delta X between 2 fiducial marks"
          # "after NL"
          # "after SL"
          # "NL line"
          # "rotation"
          n132 = call "Joystick and Camera SHIH VPC- external Connection.vi"("Motion in"=w485, "XYZTheta"=dbl[] [587.6501861346682, 659.8354057217969, 70.1155335060548, 0.010000094994154989] ("N chip"), "Measurement Point"="north chip", "Inital GO"=TRUE) -> ("Motion out"=w482:refnum<class "Motion.lvclass">, "Sum"=w462:dbl[])  [unwired: 3 in, 2 out]
          "N chip" <- w462
          n133 = call "Joystick and Camera SHIH VPC- external Connection.vi"("Motion in"=w482, "XYZTheta"=dbl[] [614.8404990206996, 1158.7590823829282, 70.34521582498871, 0.010000670236950445] ("S chip"), "Measurement Point"="south chip", "Inital GO"=TRUE) -> ("Motion out"=w481:refnum<class "Motion.lvclass">, "Sum"=w463:dbl[])  [unwired: 3 in, 2 out]
          "S chip" <- w463
          n134 = Subtract(x=w463, y=w462) -> (x-y=w461:dbl[])
          n135 = Index Array(array=w461, index #1=0 ("index"), index #2=1 ("index")) -> (element #1=w458:dbl, element #2=w457:dbl)
          n136 = Square(x=w458) -> (x^2=w455:dbl)
          n137 = Square(x=w457) -> (x^2=w456:dbl)
          n138 = Add(x=w455, y=w456) -> (x+y=w454:dbl)
          n139 = call "Joystick and Camera SHIH VPC- external Connection.vi"("Motion in"=w481, "Measurement Point"="height of stave", "Inital GO"=FALSE) -> ("Motion out"=w472:refnum<class "Motion.lvclass">, "Sum"=w473:dbl[])  [unwired: 4 in, 2 out]
          n140 = call "O to G peek.vi"("height"=w473, "south chip"=w463, "north chip"=w462, "Input file"=w474) -> ("OGP length"=→"chip distance by OGP":dbl, "output BR"=w476:dbl[], "output BL"=w475:dbl[], "output TL"=w469:dbl[])  [unwired: 4 in]
          "after NL" <- w469
          "after SR" <- w476
          "after SL" <- w475
          n141 = Square Root(x=w454) -> (sqrt(x)=→"chip distance by gantry":dbl)
          n142 = Subtract(x=w476, y=w469) -> (x-y=w487:dbl[])
          n143 = Build Array(24.3 ("y"), 231.4 ("y"), 0.0 ("element"), -0.05 ("element")) -> ()  [unwired: 1 out]
          n144 = Subtract(x=w475, y=w469) -> (x-y=w493:dbl[])
          n145 = call "XY_to_Rotation_RPHI.vi"("X-Y"=w493) -> ("r-phi"=w492:dbl[])
          n146 = Index Array(array=w492, index=1) -> (element=w489:dbl)
          n147 = Multiply(x=w489, y=-1.0) -> (x*y=w467:dbl)
          n148 = Replace Array Subset(array=w487, new element=w467, index=3) -> (→"bless from OGP !! measured stave size":dbl[])
          n149 = Replace Array Subset(array=w469, new element=w467, index=3) -> (w465:dbl[])
          n150 = Add(x=w476, y=w469) -> (x+y=w499:dbl[])
          n151 = Divide(x=w499, y=2.0) -> (x/y=w451:dbl[])
          n152 = Add(x=w465, y=dbl[] [0.0, 10.0, 0.0, 0.0]) -> (x+y=w464:dbl[])
          n153 = Replace Array Subset(array=w451, new element=w467, index=3) -> (w450:dbl[])
          "bless from OGP !!! Center of  stave" <- w450
        }
        n154 = Build Array(0.0 ("element"), 238.0 ("element"), 0.0 ("element"), 0.0 ("element")) -> (w407:dbl[])
        n155 = Add(x=w406, y=w407) -> (x+y=w405:dbl[])
        n156 = Build Array(w406, w405) -> (w404:dbl[][])
        n157 = disable-structure shown="Disabled" {
          disable-tunnel: w399 -> [w427 _]
          frame Disabled {
            # "center of lower module"
            # "center of upper module"
            n158 = Build Array(17.0 ("element"), 60.9 ("element"), 0.0 ("element"), 0.0 ("element")) -> (w429:dbl[])
            n159 = Build Array(17.0 ("element"), 411.0 ("element"), 0.0 ("element"), 0.0 ("element")) -> (w428:dbl[])
            n160 = case shown="True" w427 {
              tunnel: w429 -> [w440 w443]
              tunnel: w428 -> [w439 w442]
              tunnel: [w438 w441] -> _
              frame False {
                n161 = Build Array(w439, w440) -> (w438:dbl[][])
              }
              frame True {
                n162 = Build Array(w443, w442) -> (w441:dbl[][])
              }
            }
          }
          frame Enabled {
          }
        }
        n163 = Build Array(0.0 ("element"), 175.05 ("element"), 0.0 ("element"), 0.0 ("element")) -> (w389:dbl[])
        n164 = Build Array(0.0 ("element"), -175.05 ("element"), 0.0 ("element"), 0.0 ("element")) -> (w390:dbl[])
        n165 = case shown="False" w399 {
          tunnel: w390 -> [w446 w449]
          tunnel: w389 -> [w445 w448]
          tunnel: [w444 w447] -> w387
          frame False {
            n166 = Build Array(w445, w446) -> (w444:dbl[][])
          }
          frame True {
            n167 = Build Array(w449, w448) -> (w447:dbl[][])
          }
        }
        n168 = for {
          tunnel: w387 -> [w509] mode=indexing
          tunnel: w414 -> [w506]
          tunnel: [w508] -> w400 mode=indexing
          tunnel: w388 -> [w502]
          tunnel: [w501] -> w386 mode=indexing
          n169 = Multiply(x=w506, y=-1.0) -> (x*y=w505:dbl)
          n170 = Index Array(array=w509, index=0) -> (element=w512:dbl)
          n171 = Index Array(array=w509, index=1) -> (element=w511:dbl)
          n172 = call-poly <vilib>:"2D Cartesian Coordinate Rotation.vi"("theta"=w505, "y"=w511, "x"=w512) -> ("y out"=w514:dbl, "x out"=w513:dbl)  [unwired: 6 in, 1 out]
          n173 = Build Array(w513, w514, 0.0 ("element"), 0.0 ("element")) -> (w501:dbl[])
          n174 = Add(x=w501, y=w502) -> (x+y=w508:dbl[])
        }
        "HPoS_CT" <- w386
        n175 = Add(x=w400, y=w385) -> (x+y=w384:dbl[][])
        n176 = call-poly <vilib>:"Write Delimited Spreadsheet.vi"("file path (dialog if empty)"=path "D:/INTT/V1/Assembly Data/ladder assembly/2line_switch.txt", "format (%.3f)"="%.10f", "2D data"=w384) -> ()  [unwired: 11 in, 2 out]
      }
      event "txt switch": Value Change {
        n177 = event-data() -> ()  [unwired: 1 in, 6 out]
        n178 = flat-sequence {
          tunnel: [w537] -> w531
          tunnel: w521 -> [w533]
          tunnel: [w533] -> w520
          tunnel: w518 -> [w532]
          tunnel: [w532] -> w517
          tunnel: w531 -> [w555]
          tunnel: [w553] -> w519
          tunnel: w520 -> [w553]
          tunnel: [w552] -> w516
          tunnel: w517 -> [w552]
          frame #0 {
            n179 = call-poly <vilib>:"Read Delimited Spreadsheet.vi"("file path (dialog if empty)"=path "D:/INTT/V1/Assembly Data/ladder assembly/2line_switch.txt" ("file path (dialog if empty) 3"), "format (%.3f)"="%.10f") -> ("all rows"=w538:dbl[][])  [unwired: 8 in, 5 out]
            n180 = Array Subset(array=w538, index (row)=0 ("index"), length (row)=1 ("length"), index (col)=0 ("index"), length (col)=4 ("length")) -> (w548:dbl[][])
            n181 = Reshape Array(w548, 4 ("dimension size")) -> (w535:dbl[])
            n182 = Array Subset(array=w538, index (row)=1 ("index"), length (row)=1 ("length"), index (col)=0 ("index"), length (col)=4 ("length")) -> (w542:dbl[][])
            n183 = Reshape Array(w542, 4 ("dimension size")) -> (w536:dbl[])
            n184 = Build Array(w536, w535) -> (w537:dbl[][])
          }
          frame #1 {
            n185 = call-poly <vilib>:"Write Delimited Spreadsheet.vi"("file path (dialog if empty)"=path "D:/INTT/V1/Assembly Data/ladder assembly/2line_switch.txt" ("file path (dialog if empty) 4"), "format (%.3f)"="%.10f", "2D data"=w555) -> ()  [unwired: 11 in, 2 out]
          }
        }
      }
      event "Measure Pickup Tools": Value Change {
        (unwired) "Measuring Pickup Tools" ("String")
        n186 = event-data() -> ()  [unwired: 1 in, 6 out]
        n187 = for {
          N: w557 -> [_]
          tunnel: [w593] -> w568 mode=indexing
          tunnel: w569 -> [w597]
          tunnel: [w579] -> w567
          tunnel: w566 -> [w578] mode=indexing
          # "Default size and\norientation"
          n188 = call "Joystick and Camera SHIH VPC- external Connection.vi"("Motion in"=w597, "XYZTheta"=w578, "Measurement Point"="PickUp tool Top") -> ("Motion out"=w573:refnum<class "Motion.lvclass">, "Sum"=w596:dbl[])  [unwired: 4 in, 2 out]
          n189 = Build Array(0.0 ("element"), 29.94 ("element"), 0.0 ("element"), 0.0 ("element")) -> (w584:dbl[])
          n190 = Add(x=w596, y=w584) -> (x+y=w570:dbl[])
          n191 = Array Subset(array=w570, index=0, length=2) -> (w571:dbl[])
          n192 = call-dynamic "XY Go.vi"("Speed"=20.0, "XY"=w571, "Motion in"=w573) -> ("Motion out"=w572:refnum<class "Motion.lvclass">)  [unwired: 7 in, 1 out]
          n193 = call "Joystick and Camera SHIH VPC- external Connection.vi"("Motion in"=w572, "Measurement Point"="PickUp tool Bottom", "Inital GO"=FALSE) -> ("Motion out"=w579:refnum<class "Motion.lvclass">, "Sum"=w595:dbl[])  [unwired: 4 in, 2 out]
          n194 = Add(x=w596, y=w595) -> (x+y=w602:dbl[])
          n195 = Subtract(x=w595, y=w596) -> (x-y=w594:dbl[])
          n196 = Divide(x=w602, y=2.0) -> (x/y=w599:dbl[])
          n197 = call "XYtoRPHI.vi"("X-Y"=w594) -> ("r-phi"=w600:dbl[])
          n198 = Index Array(array=w600, index=1) -> (element=w588:dbl)
          n199 = Absolute Value(x=w588) -> (abs(x)=w591:dbl)
          n200 = Sign(1:w588) -> (0:w589:dbl)
          n201 = Subtract(x=w591, y=1.5707963267948966) -> (x-y=w590:dbl)
          n202 = Multiply(x=w589, y=w590) -> (x*y=w587:dbl)
          n203 = Replace Array Subset(array=w599, new element=w587, index=3) -> (w593:dbl[])
          "PickupTool \nCenterPosition" <- w593
        }
      }
      event "Deposit Glue": Value Change {
        # "CF height"
        # "surface z offset"
        # "two sensor, Sensor B then A"
        # "Unmount syringe"
        # "first needle park position\nneedle gap on Z value : 0.5 mm"
        # "Syringe-camera offset"
        n204 = event-data() -> ()  [unwired: 1 in, 6 out]
        n205 = call-poly <vilib>:"Read Delimited Spreadsheet.vi"("file path (dialog if empty)"=path "D:/INTT/V1/Assembly Data/Tool Offsets/Dispense Tip Offset.txt", "number of rows (all:-1)"=-1) -> ("first row"=w659:dbl[])  [unwired: 8 in, 5 out]
        n206 = Add(x=14.2 ("element"), y=w615) -> (x+y=w609:dbl)
        n207 = Index Array(array=w659, index #1=0 ("index"), index #2=1 ("index")) -> (element #1=w654:dbl, element #2=w652:dbl)
        n208 = Build Array(w654, w652, 0.0 ("element"), 0.0 ("element")) -> (w638:dbl[])
        n209 = Array Subset(array=w605, index (row)=0, length (row)=1 ("length")) -> (w618:dbl[][])  [unwired: 2 in]
        n210 = Reshape Array(w618, 4 ("dimension size")) -> (w611:dbl[])
        n211 = Index Array(array=w611, index=2) -> (element=w606:dbl)
        n212 = Add(x=w606, y=w609) -> (x+y=w608:dbl)
        n213 = Build Array(436.638, 1040.76, w608, 0.0 ("element")) -> (w607:dbl[])
        "Needle parking position" <- w607
        n214 = call "XYZTheta Go.vi"("XYZTheta In"=w607, "Motion in"=w643) -> ("error out"=w651:errorcluster, "Motion out"=w642:refnum<class "Motion.lvclass">)  [unwired: 7 in, 1 out]
        n215 = call "Display Message to User"("error in (no error)"=w651) -> ("error out"=w644:errorcluster)  [unwired: 9 in, 1 out]
        n216 = case shown="False" w613 {
          tunnel: w605 -> [w667 w676]
          tunnel: [w664 w676] -> w612
          frame False {
            n217 = Array Subset(array=w667, index (row)=1 ("index"), length (row)=1 ("length")) -> (w668:dbl[][])  [unwired: 2 in]
            n218 = Array Subset(array=w667, index (row)=0 ("index"), length (row)=1 ("length")) -> (w671:dbl[][])  [unwired: 2 in]
            n219 = Reshape Array(w671, 4 ("dimension size")) -> (w666:dbl[])
            n220 = Reshape Array(w668, 4 ("dimension size")) -> (w665:dbl[])
            n221 = Build Array(w665, w666) -> (w664:dbl[][])
          }
          frame True {
          }
        }
        n222 = call-dynamic "Z Go.vi"("error in (no error)"=w644, "Speed"=20.0, "Position"=0.0, "Motion in"=w642) -> ("error out"=w641:errorcluster, "Motion out"=w647:refnum<class "Motion.lvclass">)  [unwired: 6 in]
        n223 = call "Display Message to User2"("error in (no error)"=w641) -> ("error out"=w640:errorcluster)  [unwired: 9 in, 1 out]
        n224 = Add(x=w606, y=-2.5) -> (x+y=w648:dbl)
        n225 = call-dynamic "Z Go.vi"("error in (no error)"=w640, "Speed"=20.0, "Position"=w648, "Motion in"=w647) -> ("error out"=w617:errorcluster, "Motion out"=w639:refnum<class "Motion.lvclass">)  [unwired: 6 in]
        n226 = call-dynamic "Connect.vi"("Ultimus V in"=refnum<class "Ultimus V2.lvclass"> refnum ("Ultimus V2.lvclass")) -> ("Ultimus V out"=w637:refnum<class "Ultimus V2.lvclass">)  [unwired: 9 in, 1 out]
        n227 = for {
          N: w632 -> [_]
          tunnel: w639 -> [w691]
          tunnel: w637 -> [w690]
          tunnel: w638 -> [w692]
          tunnel: w612 -> [w693] mode=indexing
          tunnel: [w689] -> w625
          tunnel: [w688] -> w624
          tunnel: w617 -> [w684]
          tunnel: [w685] -> w616
          tunnel: w614 -> [w683]
          (unwired) 100.0 ("Speed")
          n228 = Add(x=w693, y=w692) -> (x+y=w723:dbl[])
          n229 = Add(x=w723, y=dbl[] [3.3, 5.0, 0.0, 0.0]) -> (x+y=w724:dbl[])
          n230 = Index Array(array=w724, index=2) -> (element=w681:dbl)
          n231 = Array Subset(array=w724, index=0, length=2) -> (w699:dbl[])
          n232 = call-dynamic "XY Go.vi"("error in (no error)"=w684, "Speed"=100.0, "XY"=w699, "Motion in"=w691) -> ("error out"=w679:errorcluster, "Motion out"=w680:refnum<class "Motion.lvclass">)  [unwired: 6 in]
          n233 = case shown="True" "check height?" {
            tunnel: w681 -> [_ w740]
            tunnel: w680 -> [w733 w739]
            tunnel: w679 -> [w734 w738]
            tunnel: [w734 w736] -> w678
            tunnel: [w733 w735] -> w677
            frame False {
            }
            frame True {
              n234 = call-dynamic "Z Go.vi"("error in (no error)"=w738, "Speed"=5.0, "Position"=w740, "Motion in"=w739) -> ("error out"=w737:errorcluster, "Motion out"=w735:refnum<class "Motion.lvclass">)  [unwired: 6 in]
              n235 = call "Display Message to User4"("error in (no error)"=w737) -> ("error out"=w736:errorcluster)  [unwired: 9 in, 1 out]
            }
          }
          n236 = Add(x=w681, y=-2.0) -> (x+y=w698:dbl)
          n237 = call-dynamic "Z Go.vi"("error in (no error)"=w678, "Speed"=5.0, "Position"=w698, "Motion in"=w677) -> ("error out"=w696:errorcluster, "Motion out"=w697:refnum<class "Motion.lvclass">)  [unwired: 6 in]
          n238 = call "Muliti_XY_dispense.vi"("Pressure"=w683, "Path count"=4, "distances"=dbl[][] [[0.0, 224.0], [27.4, 0.0], [0.0, -224.0], [-27.4, 0.0]], "Ultimus V in"=w690, "Motion in"=w697) -> ("Ultimus V out"=w717:refnum<class "Ultimus V2.lvclass">, "Motion out"=w722:refnum<class "Motion.lvclass">)  [unwired: 5 in]
          n239 = call-dynamic "wrtCurrent Go.vi"("axis names"=string[] ["X", "Y"], "error in (no error)"=w696, "Speed"=5.0, "distances"=dbl[] [4.6, 5.0], "Motion in"=w722) -> ("error out"=w687:errorcluster, "Motion out"=w716:refnum<class "Motion.lvclass">)  [unwired: 5 in]
          n240 = call "Muliti_XY_dispense.vi"("Pressure"=w683, "Path count"=4, "distances"=dbl[][] [[0.0, 214.0], [18.2, 0.0], [0.0, -214.0], [-18.2, 0.0]], "Ultimus V in"=w717, "Motion in"=w716) -> ("Ultimus V out"=w709:refnum<class "Ultimus V2.lvclass">, "Motion out"=w708:refnum<class "Motion.lvclass">)  [unwired: 5 in]
          n241 = call-dynamic "wrtCurrent Go.vi"("axis names"=string[] ["X", "Y"], "error in (no error)"=w687, "Speed"=5.0, "distances"=dbl[] [4.6, 5.0], "Motion in"=w708) -> ("error out"=w686:errorcluster, "Motion out"=w707:refnum<class "Motion.lvclass">)  [unwired: 5 in]
          n242 = call "Muliti_XY_dispense.vi"("Pressure"=w683, "Path count"=4, "distances"=dbl[][] [[0.0, 204.0], [9.0, 0.0], [0.0, -204.0], [-9.0, 0.0]], "Ultimus V in"=w709, "Motion in"=w707) -> ("Ultimus V out"=w694:refnum<class "Ultimus V2.lvclass">, "Motion out"=w695:refnum<class "Motion.lvclass">)  [unwired: 5 in]
          n243 = call-dynamic "wrtCurrent Go.vi"("axis names"=string[] ["X", "Y"], "error in (no error)"=w686, "Speed"=5.0, "distances"=dbl[] [4.5, 5.0], "Motion in"=w695) -> ("error out"=w685:errorcluster, "Motion out"=w701:refnum<class "Motion.lvclass">)  [unwired: 5 in]
          n244 = call "Muliti_XY_dispense.vi"("Pressure"=w683, "Path count"=1, "distances"=dbl[][] [[0.0, 194.0], [7.0, 0.0], [0.0, -206.0], [-7.0, 0.0]], "Ultimus V in"=w694, "Motion in"=w701) -> ("Ultimus V out"=w688:refnum<class "Ultimus V2.lvclass">, "Motion out"=w689:refnum<class "Motion.lvclass">)  [unwired: 5 in]
        }
        n245 = call "XYZTheta Go.vi"("error in (no error)"=w616, "XYZTheta In"=dbl[] [500.0, 1000.0, 0.0, 0.1], "Motion in"=w625) -> ("error out"=w635:errorcluster, "Motion out"=w633:refnum<class "Motion.lvclass">)  [unwired: 6 in, 1 out]
        n246 = call "Display Message to User3"("error in (no error)"=w635) -> ()  [unwired: 9 in, 2 out]
        n247 = call-dynamic "Disconnect.vi"("Ultimus V in"=w624) -> ()  [unwired: 9 in, 1 out]
      }
      event "Needle Alignment": Value Change {
        (unwired) "Needle Alignment in progress ...." ("String")
        # "CF height"
        # "surface z offset"
        # "first needle park position\nneedle gap on Z value : 0.5 mm"
        # "Syringe-camera offset"
        n248 = event-data() -> ()  [unwired: 1 in, 6 out]
        n249 = Array Subset(array=w744, index (row)=0, length (row)=1 ("length")) -> (w747:dbl[][])  [unwired: 2 in]
        n250 = Reshape Array(w747, 4 ("dimension size")) -> (w746:dbl[])
        n251 = Index Array(array=w746, index=2) -> (element=w743:dbl)
        n252 = call-poly <vilib>:"Read Delimited Spreadsheet.vi"("file path (dialog if empty)"=path "D:/INTT/V1/Assembly Data/Tool Offsets/Dispense Tip Offset.txt", "number of rows (all:-1)"=-1) -> ("first row"=w794:dbl[])  [unwired: 8 in, 5 out]
        n253 = Index Array(array=w794, index #1=0 ("index"), index #2=1 ("index")) -> (element #1=w789:dbl, element #2=w788:dbl)
        n254 = Add(x=14.2 ("element"), y=w752) -> (x+y=w754:dbl)
        n255 = Add(x=w743, y=w754) -> (x+y=w753:dbl)
        n256 = Build Array(436.638, 1040.76, w753, 0.0 ("element")) -> (w751:dbl[])
        n257 = Build Array(w789, w788, 0.0 ("element"), 0.0 ("element")) -> (w763:dbl[])
        n258 = call "XYZTheta Go.vi"("XYZTheta In"=w751, "Motion in"=w778) -> ("error out"=w787:errorcluster, "XYZTheta Out"=w768:dbl[], "Motion out"=w777:refnum<class "Motion.lvclass">)  [unwired: 7 in]
        n259 = call "Display Message to User10"("error in (no error)"=w787) -> ("error out"=w784:errorcluster)  [unwired: 9 in, 1 out]
        n260 = call-dynamic "Z Go.vi"("error in (no error)"=w784, "Speed"=20.0, "Position"=0.0, "Motion in"=w777) -> ("Motion out"=w776:refnum<class "Motion.lvclass">)  [unwired: 6 in, 1 out]
        n261 = Replace Array Subset(array=w768, new element=0.0 ("new element/subarray"), index=2) -> (w765:dbl[])
        n262 = call "Joystick and Camera - external Connection.vi"("Motion in"=w776, "XYZTheta"=w765, "Measurement Point"="Touch Needle on a surface") -> ("Motion out"=w774:refnum<class "Motion.lvclass">, "Gantry"=w764:dbl[])  [unwired: 4 in, 2 out]
        n263 = Subtract(x=w764, y=w763) -> (x-y=w762:dbl[])
        n264 = call "Joystick and Camera - external Connection.vi"("Motion in"=w774, "XYZTheta"=w762, "Measurement Point"="Measure the touch spot with camera") -> ("Motion out"=w770:refnum<class "Motion.lvclass">, "Gantry"=w773:dbl[])  [unwired: 4 in, 2 out]
        n265 = Subtract(x=w764, y=w773) -> (x-y=w772:dbl[])
        n266 = call-poly <vilib>:"Write Delimited Spreadsheet.vi"("file path (dialog if empty)"=path "D:/INTT/V1/Assembly Data/Tool Offsets/Dispense Tip Offset.txt", "1D data"=w772, "append to file? (new file:F)"=FALSE) -> ()  [unwired: 11 in, 2 out]
      }
      event "Pick and place": Value Change {
        (unwired) "PICK and PLACE samples ..." ("String")
        n267 = event-data() -> ()  [unwired: 1 in, 6 out]
        n268 = Build Array(0.0 ("element"), 58.4 ("element"), 0.0 ("element"), 0.0 ("element")) -> (w803:dbl[])
        n269 = Build Array(0.0 ("element"), -58.4 ("element"), 0.0 ("element"), 0.0 ("element")) -> (w802:dbl[])
        n270 = case shown="False" w818 {
          tunnel: w824 -> [w966 w988]
          tunnel: [w965 w987] -> _
          frame False {
            n271 = Array Subset(array=w966, index (row)=0 ("index"), length (row)=1 ("length")) -> (w968:dbl[][])  [unwired: 2 in]
            n272 = Build Array(11.75 ("element"), 173.55 ("element"), 0.0 ("element"), 0.0 ("element")) -> (w972:dbl[])
            n273 = Reshape Array(w968, 4 ("dimension size")) -> (w967:dbl[])
            n274 = Add(x=w972, y=w967) -> (x+y=w965:dbl[])
          }
          frame True {
            n275 = Array Subset(array=w988, index (row)=0 ("index"), length (row)=1 ("length")) -> (w978:dbl[][])  [unwired: 2 in]
            n276 = Build Array(11.75 ("element"), 56.85 ("element"), 0.0 ("element"), 0.0 ("element")) -> (w982:dbl[])
            n277 = Reshape Array(w978, 4 ("dimension size")) -> (w977:dbl[])
            n278 = Add(x=w982, y=w977) -> (x+y=w987:dbl[])
          }
        }
        n279 = case shown="False" w818 {
          tunnel: w803 -> [w959 w962]
          tunnel: w802 -> [w960 w963]
          tunnel: [w961 w964] -> w801
          frame False {
            n280 = Build Array(w960, w959) -> (w961:dbl[][])
          }
          frame True {
            n281 = Build Array(w962, w963) -> (w964:dbl[][])
          }
        }
        n282 = for {
          tunnel: [w846] -> w817
          tunnel: w801 -> [w845] mode=indexing
          n283 = Index Array(array=w845, index=3) -> (element=w843:dbl)
          n284 = Multiply(x=w843, y=-1.0) -> ()  [unwired: 1 out]
          n285 = Index Array(array=w845, index=0) -> (element=w852:dbl)
          n286 = Index Array(array=w845, index=1) -> (element=w851:dbl)
          n287 = call-poly <vilib>:"2D Cartesian Coordinate Rotation.vi"("theta"=w843, "y"=w851, "x"=w852) -> ("y out"=w854:dbl, "x out"=w853:dbl)  [unwired: 6 in, 1 out]
          n288 = Build Array(w853, w854, 0.0 ("element"), 0.0 ("element")) -> (w846:dbl[])
        }
        n289 = Array Subset(array=w799, index (row)=0 ("index"), length (row)=1 ("length")) -> (w809:dbl[][])  [unwired: 2 in]
        n290 = Reshape Array(w809, 4 ("dimension size")) -> (w800:dbl[])
        n291 = Add(x=w817, y=w800) -> (x+y=w798:dbl[])
        "x+y" <- w798
        n292 = call-poly <vilib>:"Read Delimited Spreadsheet.vi"("file path (dialog if empty)"=path "D:/INTT/V1/Assembly Data/Tool Offsets/Bellows Tool Offset.txt", "number of rows (all:-1)"=-1) -> ("first row"=w839:dbl[])  [unwired: 8 in, 5 out]
        n293 = Index Array(array=w839, index #1=0 ("index"), index #2=1 ("index"), index #3=2 ("index")) -> (element #1=w835:dbl, element #2=w834:dbl, element #3=w833:dbl)
        n294 = for {
          N: 1 -> [_]
          tunnel: w842 -> [w864]
          tunnel: [w885] -> w832
          tunnel: w831 -> [w857] mode=indexing
          tunnel: [w873] -> w827
          tunnel: w828 -> [w863]
          tunnel: w835 -> [w887]
          tunnel: w834 -> [w886]
          tunnel: w833 -> [w884]
          tunnel: w820 -> [w879]
          tunnel: w826 -> [w866]
          tunnel: w798 -> [w865]
          tunnel: w822 -> [w861]
          tunnel: w799 -> [w856]
          w875 = 0 ("Write")
          w878 = TRUE ("Write Value")
          # "putback pickup tool"
          # "pickup tool"
          # "pickup tool height offset"
          # "Pick up PICKUP TOOL"
          # "Pick up CHIPs/Sensor and place on HDI"
          n295 = Build Array(w887, w886, w884, 0.0 ("element")) -> (w858:dbl[])
          n296 = Add(x=w857, y=w858) -> (x+y=w859:dbl[])
          n297 = call "XYZTheta-2Zspeed Go.vi"("XYZTheta In"=w859, "Motion in"=w864) -> ("error out"=w862:errorcluster, "Motion out"=w860:refnum<class "Motion.lvclass">)  [unwired: 7 in, 1 out]
          n298 = call "WriteReadWait.vi"("Read Value"=w878, "Write Value"=w878, "error in (no error)"=w862, "Read"=w875, "Write"=w875, "I-O in"=w863) -> ("error out"=w877:errorcluster, "I-O out"=w876:refnum<class "NI-DAQ.lvclass">)  [unwired: 4 in]
          n299 = Replace Array Subset(array=w858, new element=-16.0 ("t"), index=2) -> (w882:dbl[])
          n300 = for {
            N: w879 -> [_]
            tunnel: w860 -> [w906]
            tunnel: w882 -> [w905]
            tunnel: w877 -> [w904]
            tunnel: [w903] -> w888
            tunnel: w876 -> [w902]
            tunnel: [w901] -> w874
            tunnel: [w900] -> w881
            tunnel: w866 -> [w897]
            tunnel: w865 -> [w894]
            tunnel: w861 -> [w896] mode=indexing
            tunnel: w856 -> [w895] mode=indexing
            n301 = flat-sequence {
              tunnel: [w926] -> w907
              tunnel: w906 -> [w925]
              tunnel: w905 -> [w924]
              tunnel: w904 -> [w922]
              tunnel: w902 -> [w914]
              tunnel: [w921] -> w899
              tunnel: [w918] -> w898
              tunnel: w897 -> [w911]
              tunnel: w894 -> [w917]
              tunnel: w907 -> [w946]
              tunnel: [w958] -> w903
              tunnel: [w957] -> _
              tunnel: [w953] -> w901
              tunnel: [w950] -> w900
              tunnel: w899 -> [w955]
              tunnel: w898 -> [w951]
              tunnel: w896 -> [w952]
              tunnel: w895 -> [_]
              tunnel: w894 -> [w927]
              frame #0 {
                w912 = FALSE ("Write Value")
                w919 = TRUE ("Write Value")
                w920 = 1 ("Write")
                # "pickup module"
                # "release module"
                # "pickup sample from tray"
                n302 = Add(x=w917, y=w924) -> (x+y=w923:dbl[])
                n303 = call "XYZTheta-2Zspeed Go.vi"("error in (no error)"=w922, "XYZTheta In"=w923, "Motion in"=w925) -> ("error out"=w915:errorcluster, "Motion out"=w926:refnum<class "Motion.lvclass">)  [unwired: 6 in, 1 out]
                n304 = call "Time Delay"("error in (no error)"=w915) -> ("error out"=w908:errorcluster)  [unwired: 10 in]
                n305 = call "0"("error in (no error)"=w908) -> ("error out"=w909:errorcluster)  [unwired: 9 in, 1 out]
                n306 = call "WriteReadWait.vi"("Read Value"=w912, "Write Value"=w912, "error in (no error)"=w909, "Read"=w911, "Write"=w911, "I-O in"=w914) -> ("error out"=w910:errorcluster, "I-O out"=w913:refnum<class "NI-DAQ.lvclass">)  [unwired: 4 in]
                n307 = call "Time Delay3"("error in (no error)"=w910) -> ("error out"=w916:errorcluster)  [unwired: 10 in]
                n308 = call "WriteReadWait.vi"("Read Value"=w919, "Write Value"=w919, "error in (no error)"=w916, "Read"=w920, "Write"=w920, "I-O in"=w913) -> ("error out"=w918:errorcluster, "I-O out"=w921:refnum<class "NI-DAQ.lvclass">)  [unwired: 4 in]
              }
              frame #1 {
                w954 = 1 ("Write")
                w956 = FALSE ("Write Value")
                # "lift for chip/sensor thickness"
                # "place sample on HDI"
                n309 = Add(x=w952, y=dbl[] [0.0, 0.0, -16.0, 0.0]) -> (x+y=w944:dbl[])
                n310 = call-dynamic "Get Current Position.vi"("Motion in"=w946) -> ("XYZTheta Out"=w942:dbl[], "Motion out"=w945:refnum<class "Motion.lvclass">)  [unwired: 8 in, 1 out]
                "gantry position test" <- w942
                n311 = Array Subset(array=w927, index=0, length=2) -> (w931:dbl[])
                n312 = Build Array (concatenate)(w931, 0.0 ("element"), 0.0 ("element")) -> (w930:dbl[])
                n313 = Subtract(x=w944, y=w930) -> (x-y=w943:dbl[])
                "displacement" <- w943
                n314 = Array Subset(array=w942, index=0, length=2) -> (w937:dbl[])
                n315 = Build Array (concatenate)(w937, 0.0 ("element"), 0.0 ("element")) -> (w936:dbl[])
                n316 = Add(x=w936, y=w943) -> (x+y=w929:dbl[])
                "stave target position" <- w929
                n317 = call "XYZTheta-2Zspeed Go.vi"("error in (no error)"=w951, "XYZTheta In"=w929, "Motion in"=w945) -> ("error out"=w949:errorcluster, "XYZTheta Out"=w957:dbl[], "Motion out"=w958:refnum<class "Motion.lvclass">)  [unwired: 6 in]
                n318 = call "1"("error in (no error)"=w949) -> ("error out"=w948:errorcluster)  [unwired: 9 in, 1 out]
                n319 = call "Time Delay6"("error in (no error)"=w948) -> ("error out"=w947:errorcluster)  [unwired: 10 in]
                n320 = call "WriteReadWait.vi"("Read Value"=w956, "Write Value"=w956, "error in (no error)"=w947, "Read"=w954, "Write"=w954, "I-O in"=w955) -> ("error out"=w950:errorcluster, "I-O out"=w953:refnum<class "NI-DAQ.lvclass">)  [unwired: 4 in]
              }
            }
          }
          n321 = call "XYZTheta-2Zspeed Go.vi"("error in (no error)"=w881, "XYZTheta In"=w859, "Motion in"=w888) -> ("error out"=w869:errorcluster, "Motion out"=w892:refnum<class "Motion.lvclass">)  [unwired: 6 in, 1 out]
          n322 = call "Time Delay9"("error in (no error)"=w869) -> ("error out"=w871:errorcluster)  [unwired: 10 in]
          n323 = call-dynamic "Digital Write 1 Channel.vi"("DAQ Module"=0, "error constant"=w871, "Value"=FALSE, "Channel"=0, "NI-DAQ.lvclass"=w874) -> ("error IO"=w870:errorcluster, "NI-DAQ.lvclass 2"=w873:refnum<class "NI-DAQ.lvclass">)  [unwired: 5 in]
          n324 = call "Time Delay10"("error in (no error)"=w870) -> ("error out"=w889:errorcluster)  [unwired: 10 in]
          n325 = call-dynamic "Z Go.vi"("error in (no error)"=w889, "Speed"=10.0, "Position"=0.0 ("new element/subarray"), "Motion in"=w892) -> ("Motion out"=w885:refnum<class "Motion.lvclass">)  [unwired: 6 in, 1 out]
        }
      }
      event "GOTO": Value Change {
        (unwired) "GOING to a position" ("String")
        n326 = event-data() -> ()  [unwired: 1 in, 6 out]
        n327 = call "XYZTheta Go.vi"("XYZTheta In"="Parking position", "Motion in"=w995) -> ("Motion out"=w993:refnum<class "Motion.lvclass">)  [unwired: 7 in, 2 out]
      }
      event "READ Position": Value Change {
        n328 = event-data() -> ()  [unwired: 1 in, 6 out]
        n329 = call-dynamic "Get Current Position.vi"("Motion in"=w1014) -> ("XYZTheta Out"=→"Gantry current position":dbl[], "Motion out"=w1013:refnum<class "Motion.lvclass">)  [unwired: 8 in, 1 out]
      }
      event "HDI vacuum": Value Change {
        n330 = event-data() -> ()  [unwired: 1 in, 6 out]
        n331 = call "WriteReadWait.vi"("Read Value"="vacuum", "Write Value"="vacuum", "Read"=w1026, "Write"=w1026, "I-O in"=w1029) -> ("error out"=w1027:errorcluster, "I-O out"=w1016:refnum<class "NI-DAQ.lvclass">)  [unwired: 5 in]
        n332 = call "Time Delay2"("error in (no error)"=w1027) -> ()  [unwired: 10 in, 1 out]
      }
      event Timeout {
        n333 = event-data() -> ()  [unwired: 1 in, 3 out]
        n334 = call-dynamic "Digital Read 1 Channel.vi"("Read"=w1041, "NI-DAQ in"=w1042) -> ("Value"=→"Status":bool, "NI-DAQ out"=w1040:refnum<class "NI-DAQ.lvclass">)  [unwired: 7 in, 1 out]
      }
    }
    "Measured HDI size" <- w25
    "module positions on stave" <- w26
    "Stave mark" <- w24
    "measured HDI top-left position" <- w21
    n335 = feedback-in #1(w25) -> ()
    n336 = feedback-in #2(w24) -> ()
    n337 = feedback-in #3(w21) -> ()
    n338 = feedback-in #4(w10) -> ()
    n339 = feedback-in #5(w36) -> ()
    n340 = feedback-in #6(w33) -> ()
    n341 = feedback-in #7(w41) -> ()
    n342 = feedback-in #8(w26) -> ()
    n343 = feedback-in #9(w42) -> ()
    "# of tasks excuted" <- w38
  }
  n344 = call-dynamic "Disconnect.vi"("Controller in"=w4) -> ()  [unwired: 9 in, 1 out]
  n345 = call-dynamic "Disconnect.vi"("I-O in"=w1) -> ()  [unwired: 9 in, 1 out]
